vi "Omniax_mDrive_XYZR_MM_BR_RES.vi"() -> ()   [LabVIEW 2009]
uses:
  <vilib>/Instr/_visa.llb/VISA Configure Serial Port (Instr).vi
panel:
  out "R Backlash steps/sec":i32
  out "R Backlash":i32
  out "R Holding Current %":i32
  out "R Run Current %":i32
  out "R offset deg":dbl
  out "R deg/rev":dbl
  out "R steps/rev":u32
  out "R velocity PV step/sec":i32
  out "R MINPOS":i32=-94296
  out "R MAXPOS":i32=-34296
  out "R COM PORT":refnum<visa-resource-name>="COM5"
  in  "R Scan set":bool
  in  "R Scan Velocity SP deg/sec":dbl
  in  "R Scan Length SP deg":dbl
  in  "R Move Set":bool
  out "Reset R Motor Steps":i32
  in  "Reset R Position deg":dbl
  out "R Velocity MVdeg/sec":dbl
  in  "R Velocity SP deg/sec":dbl
  in  "R Position SP deg":dbl
  out "R Position MV deg":dbl
  out "R Scan velocity MV deg/sec":dbl format="%#_6f"
  out "R Scan length MV deg":dbl
  in  "R Scan Length SP steps":i32 min=-460800 max=460800 step=100
  in  "R Scan OK":bool
  in  "R Velocity SP step/sec":i32 min=1 max=102400
  in  "R Scan Velocity SP steps/sec":i32=1 min=1 max=102400 step=1
  in  "R Go":bool
  in  "R Step SP":i32=-20000 min=0 max=6144000 step=500
  out "R Position deg PV":dbl
  out "R Step PV":i32 max=2000
  out "R Backlash corr":bool
  out "R in Motion":bool
  out "R Scan":bool
  out "R in Range":bool
  out "Z COM PORT":refnum<visa-resource-name>="COM5"
  out "Z Backlash steps/sec":i32
  out "Z Backlash":i32
  out "Z Holding Current %":i32
  out "Z Run Current %":i32
  out "Z offset mm":dbl
  out "Z mm/rev":dbl
  out "Z steps/rev":u32
  out "Z  velocity PV step/sec":i32
  out "Z MINPOS":i32=-94296
  out "Z MAXPOS":i32=-34296
  in  "Z Scan set":bool
  in  "Z Scan Velocity SP mm/sec":dbl
  in  "Z Scan Length SP mm":dbl
  in  "Z Move Set":bool
  out "Reset Z Motor Steps":i32
  in  "Reset Z Position mm":dbl
  out "Z Velocity MV mm/sec":dbl
  in  "Z Velocity SP mm/sec":dbl
  in  "Z Position SP mm":dbl
  out "Z Position MV mm":dbl
  out "Z Scan velocity MV mm/sec":dbl format="%#_6f"
  out "Z Scan length MV mm":dbl
  in  "Z Scan Length SP steps":i32 min=-460800 max=460800 step=100
  in  "Z Scan OK":bool
  in  "Z Velocity SP step/sec":i32 min=1 max=102400
  in  "Z Scan Velocity SP steps/sec":i32=1 min=1 max=102400 step=1
  in  "Z Go":bool
  in  "Z Step SP":i32=-20000 min=0 max=2048000 step=500
  out "Z Position mm PV":dbl
  out "Z Step PV":i32 max=2000
  out "Z Backlash corr":bool
  out "Z in Motion":bool
  out "Z Scan":bool
  out "Z in Range":bool
  out "Reset X Motor Steps":i32
  in  "Reset X Position mm":dbl
  out "X Backlash corr":bool
  out "X  in Motion":bool
  out "X Scan":bool
  out "X  in Range":bool
  out "X Step PV":i32 max=2000
  out "X Position mm PV":dbl
  out "X velocity PV step/sec":i32
  in  "X Scan set":bool
  in  "X Scan Velocity SP mm/sec":dbl
  in  "X Scan Length SP mm":dbl
  in  "X Move Set":bool
  out "X Velocity MV mm/sec":dbl
  in  "X Velocity SP mm/sec":dbl
  in  "X Position SP mm":dbl
  out "X Position MV mm":dbl
  out "X Scan velocity MV mm/sec":dbl format="%#_6f"
  out "X Scan length MV mm":dbl
  in  "X Scan Length SP steps":i32 min=-460800 max=460800 step=100
  in  "X Scan OK":bool
  in  "X Velocity SP step/sec":i32 min=1 max=102400
  in  "X Scan Velocity SP steps/sec":i32=1 min=1 max=102400 step=1
  in  "X Go":bool
  in  "X Step SP":i32=-20000 min=-460800 max=460800 step=500
  out "X Backlash steps/sec":i32
  out "X Backlash":i32
  out "X Holding Current %":i32
  out "X Run Current %":i32
  out "X offset mm":dbl
  out "X mm/rev":dbl
  out "X steps/rev":u32
  out "X MAXPOS":i32=-34296
  out "X MINPOS":i32=-94296
  out "X COM PORT":refnum<visa-resource-name>="COM5"
  out "Y Backlash corr":bool
  in  "Y Scan set":bool
  in  "Y Scan Velocity SP mm/sec":dbl
  in  "Y Scan Length SP mm":dbl
  in  "Y Move Set":bool
  out "Y Backlash steps/sec":i32
  out "Y Backlash":i32
  out "Y in Motion":bool
  in  "Reset":bool
  out "Reset Y Motor Steps":i32
  in  "Reset Y Position mm":dbl
  out "Y Velocity MV mm/sec":dbl
  in  "Y Velocity SP mm/sec":dbl
  in  "Y Position SP mm":dbl
  out "Y Position MV mm":dbl
  out "Y Holding Current %":i32
  out "Y Run Current %":i32
  out "Y Scan velocity MV mm/sec":dbl format="%#_6f"
  out "Y Scan length MV mm":dbl
  in  "Scan Cancel":bool
  out "Y Position mm PV":dbl
  out "Y offset mm":dbl
  out "Y mm/rev":dbl
  out "Y steps/rev":u32
  out "Y velocity PV step/sec":i32
  in  "Y Scan Length SP steps":i32 min=-460800 max=460800 step=100
  out "Y Scan":bool
  in  "Y Scan OK":bool
  in  "Scan Go":bool
  in  "Y Velocity SP step/sec":i32 min=1 max=102400
  in  "Y Scan Velocity SP steps/sec":i32=1 min=1 max=102400 step=1
  in  "Stop":bool
  out "Y in Range":bool
  out "Y Step PV":i32 max=2000
  in  "Y Go":bool
  in  "Y Step SP":i32=-20000 min=-460800 max=460800 step=500
  out "Y MINPOS":i32=-94296
  out "Y MAXPOS":i32=-34296
  out "Y COM PORT":refnum<visa-resource-name>="COM5"
  # "LM"
  # "MV"
  # "BL"
  # "SC"
  # "MX"
  # "MY"
  # "MZ"
  # "MR"
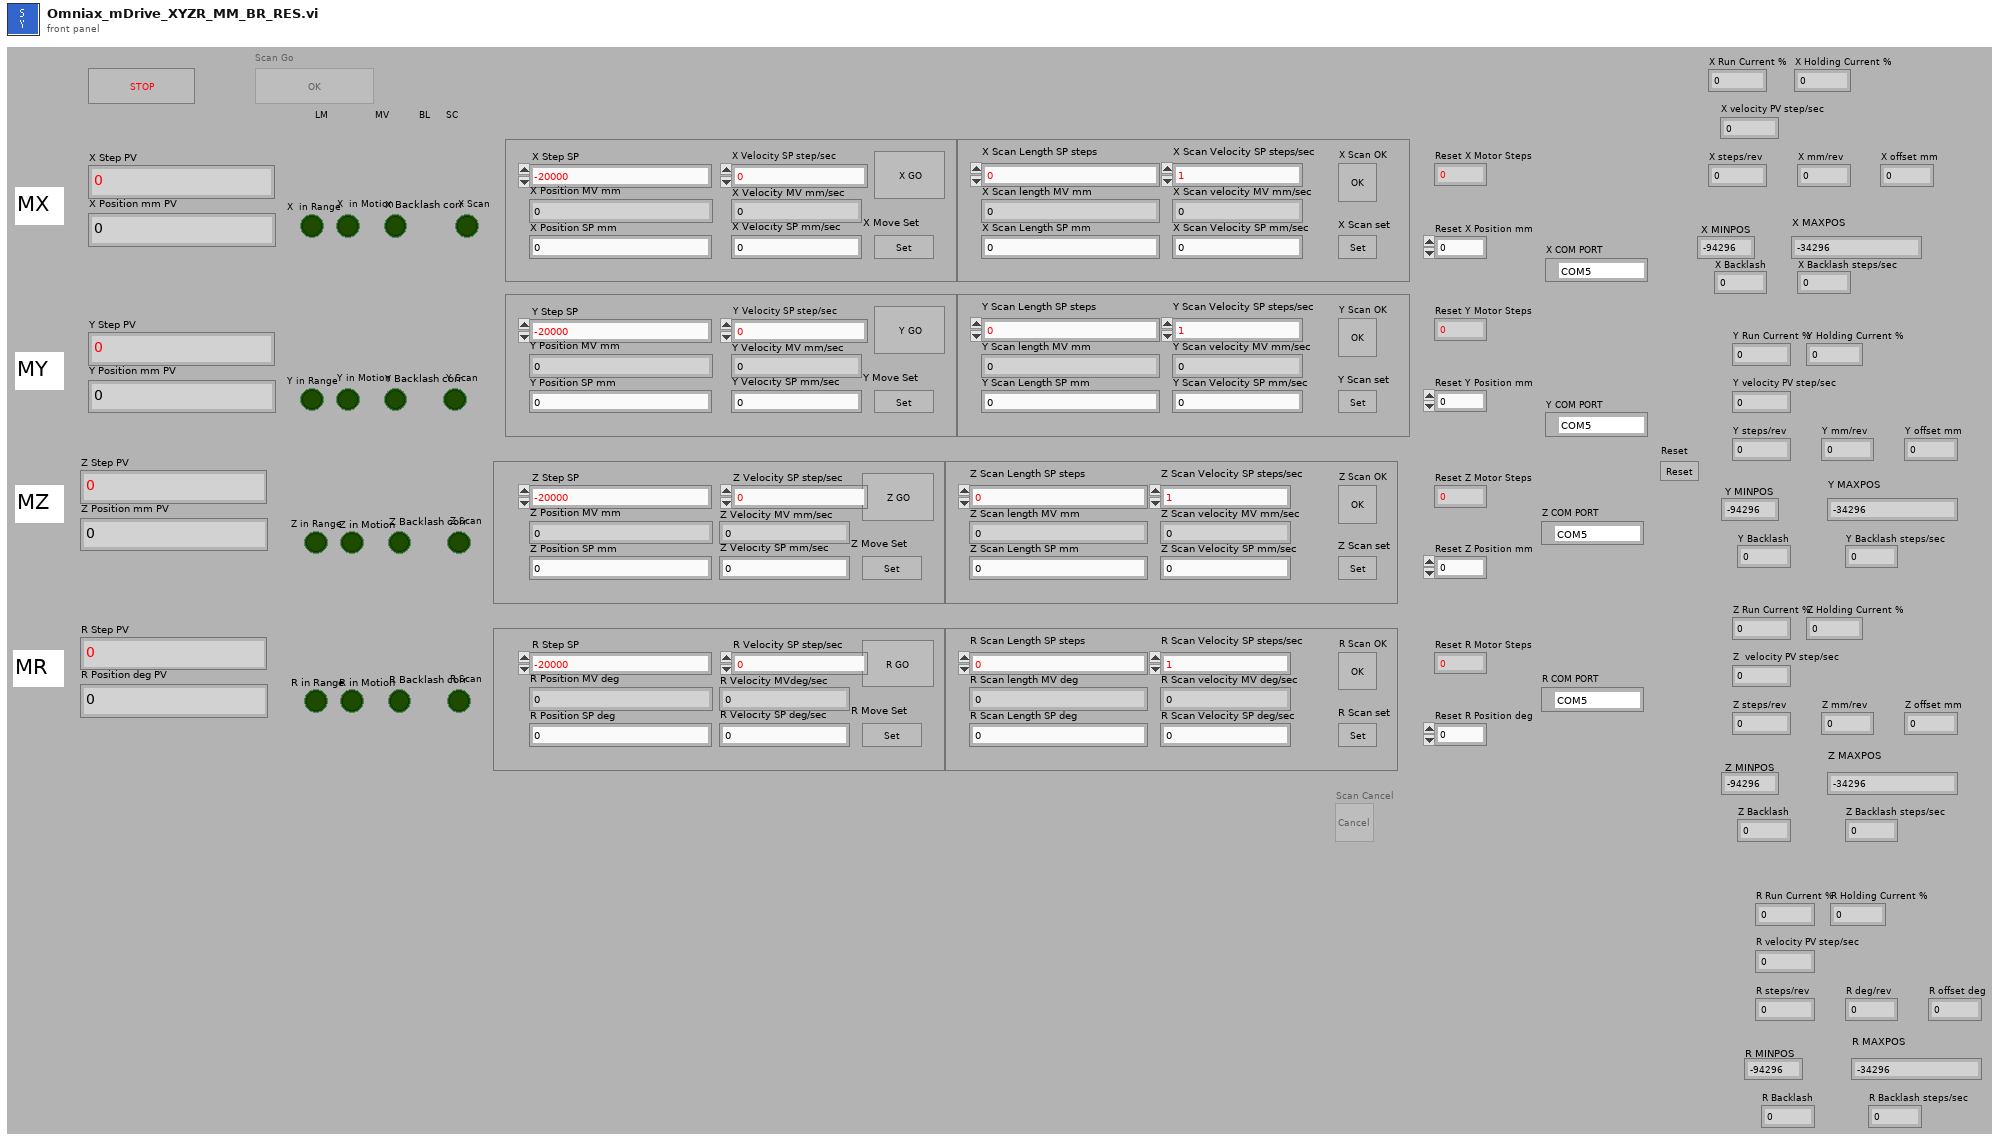
[diagram p1: front panel]
types:
  T1 = enum8{"Enabled", "Disabled", "Disabled and Grayed Out"}
  T2 = enum16{"Stop", "Reset", "Run Current", "Holding Current", "Accel Rate", "Decel Rate", "Move to Relative Position", "Move to Absolute Position", "Echo Mode", "Print Parameter", "Send String", "Microstep Resolution", "Set Current Position", "Max Velocity"}
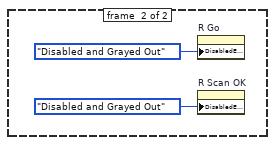
[diagram p2: hidden frame]
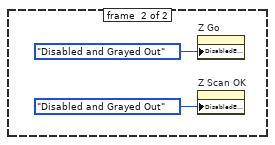
[diagram p5: hidden frame]
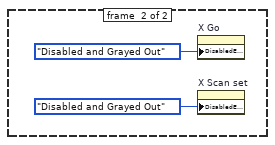
[diagram p8: hidden frame]
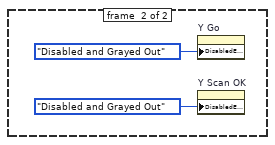
[diagram p11: hidden frame]
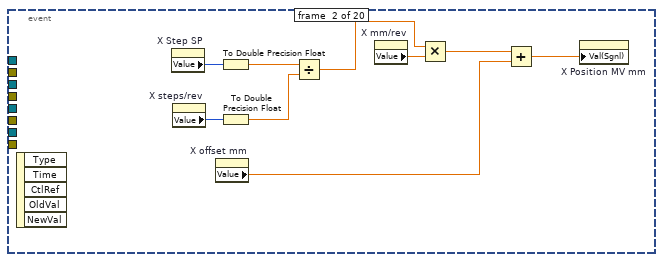
[diagram p14: hidden frame]
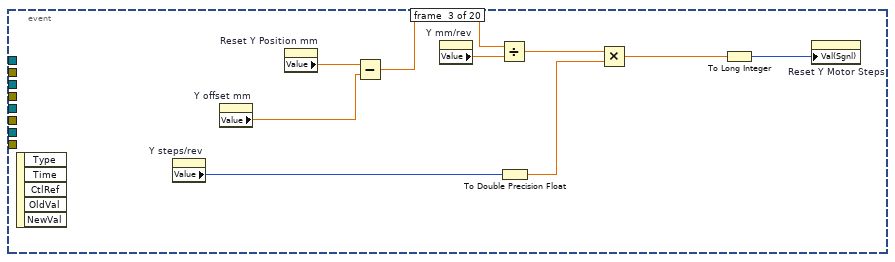
[diagram p15: hidden frame]
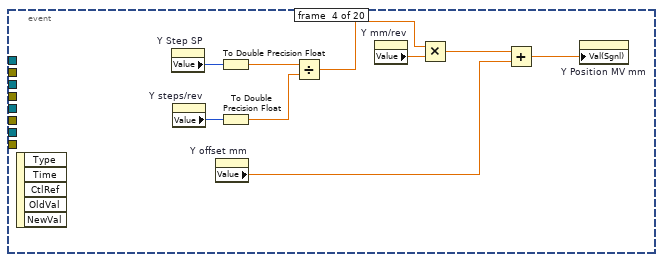
[diagram p16: hidden frame]
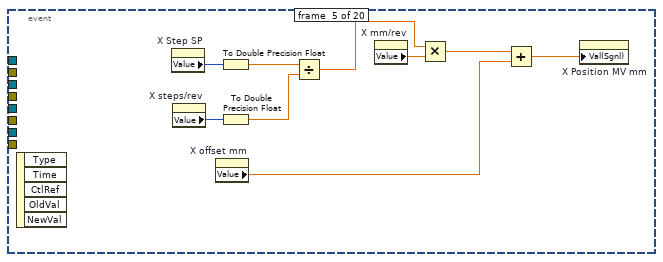
[diagram p17: hidden frame]
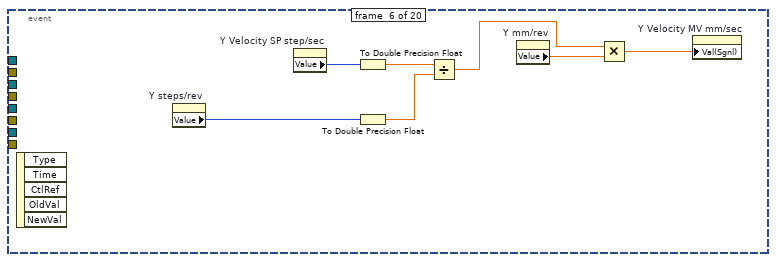
[diagram p18: hidden frame]
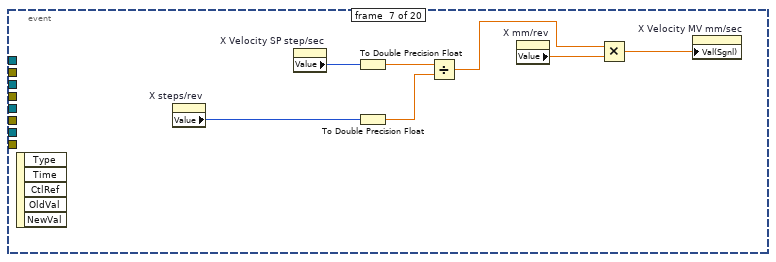
[diagram p19: hidden frame]
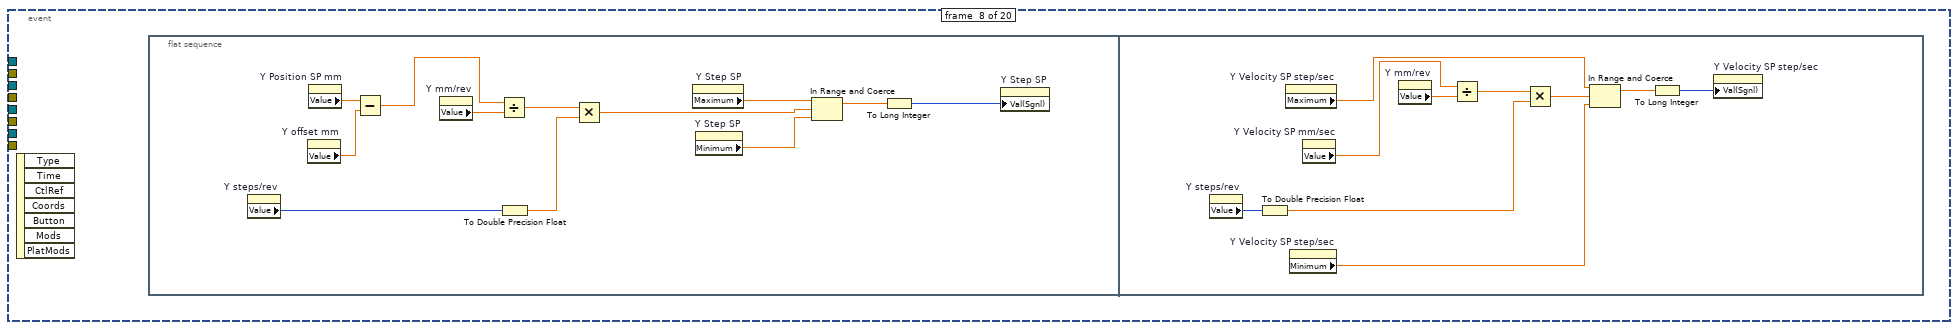
[diagram p20: hidden frame]
diagram:
  w11 = refnum<visa-resource-name> "COM11" ("COM PORT")
  w13 = u16 0 items=["None", "XON/XOFF", "RTS/CTS", "XON/XOFF & RTS/CTS", "DTR/DSR", "XON/XOFF & DTR/DSR"] ("flow control (0:none)")
  w14 = u16 10 items=["1.0"=10, "1.5"=15, "2.0"=20] ("stop bits (10: 1 bit)")
  w44 = refnum<visa-resource-name> "COM10" ("COM PORT")
  w46 = u16 0 items=["None", "XON/XOFF", "RTS/CTS", "XON/XOFF & RTS/CTS", "DTR/DSR", "XON/XOFF & DTR/DSR"] ("flow control (0:none)")
  w47 = u16 10 items=["1.0"=10, "1.5"=15, "2.0"=20] ("stop bits (10: 1 bit)")
  w57 = refnum<visa-resource-name> "COM8" ("COM PORT")
  w59 = u16 0 items=["None", "XON/XOFF", "RTS/CTS", "XON/XOFF & RTS/CTS", "DTR/DSR", "XON/XOFF & DTR/DSR"] ("flow control (0:none)")
  w60 = u16 10 items=["1.0"=10, "1.5"=15, "2.0"=20] ("stop bits (10: 1 bit)")
  w82 = refnum<visa-resource-name> "COM9" ("COM PORT")
  w84 = u16 0 items=["None", "XON/XOFF", "RTS/CTS", "XON/XOFF & RTS/CTS", "DTR/DSR", "XON/XOFF & DTR/DSR"] ("flow control (0:none)")
  w85 = u16 10 items=["1.0"=10, "1.5"=15, "2.0"=20] ("stop bits (10: 1 bit)")
  # "Stop bits"
  # "Stop bits"
  # "Stop bits"
  # "Stop bits"
  n1 = flat-sequence {
    frame #0 {
      w93 = 3.0 ("R deg/rev")
      w91 = u32 51200 ("step/rev")
      w95 = 102400 ("Value (Signaling)")
      n2 = property on="R Velocity SP step/sec" class="DigNum (strict)"("Val(Sgnl)"=w95) -> ()  [unwired: 2 in, 2 out]
      n3 = property on="R Velocity SP step/sec" class="DigNum (strict)"("Minimum"=1.0 ("Data Entry Limits:Minimum")) -> ()  [unwired: 2 in, 2 out]
      n4 = To Double Precision Float(number=w91) -> (double precision float=w92:dbl)
      n5 = To Double Precision Float(number=w95) -> (double precision float=w97:dbl)
      n6 = Divide(x=w97, y=w92) -> (x/y=w96:dbl)
      n7 = property on="R Velocity SP step/sec" class="DigNum (strict)"("Maximum"=w97) -> ()  [unwired: 2 in, 2 out]
      n8 = Multiply(x=w96, y=w93) -> (x*y=w94:dbl)
      n9 = property on="R Velocity SP deg/sec" class="DigNum (strict)"("Val(Sgnl)"=w94) -> ()  [unwired: 2 in, 2 out]
      "R offset deg" <- 0.0 ("R offset deg")
      "R deg/rev" <- w93
      "R steps/rev" <- w91
    }
  }
  n10 = flat-sequence {
    frame #0 {
      w100 = 1.0 ("MM/rev")
      w103 = u32 51200 ("step/rev")
      w98 = 102400 ("Value (Signaling)")
      n11 = property on="X Velocity SP step/sec" class="DigNum (strict)"("Minimum"=1.0 ("Data Entry Limits:Minimum")) -> ()  [unwired: 2 in, 2 out]
      n12 = property on="X Velocity SP step/sec" class="DigNum (strict)"("Val(Sgnl)"=w98) -> ()  [unwired: 2 in, 2 out]
      n13 = To Double Precision Float(number=w103) -> (double precision float=w102:dbl)
      n14 = To Double Precision Float(number=w98) -> (double precision float=w104:dbl)
      n15 = Divide(x=w104, y=w102) -> (x/y=w99:dbl)
      n16 = property on="X Velocity SP step/sec" class="DigNum (strict)"("Maximum"=w104) -> ()  [unwired: 2 in, 2 out]
      n17 = Multiply(x=w99, y=w100) -> (x*y=w101:dbl)
      n18 = property on="X Velocity SP mm/sec" class="DigNum (strict)"("Val(Sgnl)"=w101) -> ()  [unwired: 2 in, 2 out]
      "X offset mm" <- 0.0 ("offset")
      "X steps/rev" <- w103
      "X mm/rev" <- w100
    }
  }
  n19 = flat-sequence {
    frame #0 {
      w108 = 1.0 ("Z mm/rev")
      w107 = u32 51200 ("step/rev")
      w109 = 102400 ("Value (Signaling)")
      n20 = property on="Z Velocity SP step/sec" class="DigNum (strict)"("Val(Sgnl)"=w109) -> ()  [unwired: 2 in, 2 out]
      n21 = property on="Z Velocity SP step/sec" class="DigNum (strict)"("Minimum"=1.0 ("Data Entry Limits:Minimum")) -> ()  [unwired: 2 in, 2 out]
      n22 = To Double Precision Float(number=w107) -> (double precision float=w112:dbl)
      n23 = To Double Precision Float(number=w109) -> (double precision float=w113:dbl)
      n24 = Divide(x=w113, y=w112) -> (x/y=w110:dbl)
      n25 = property on="Z Velocity SP step/sec" class="DigNum (strict)"("Maximum"=w113) -> ()  [unwired: 2 in, 2 out]
      n26 = Multiply(x=w110, y=w108) -> (x*y=w111:dbl)
      n27 = property on="Z Velocity SP mm/sec" class="DigNum (strict)"("Val(Sgnl)"=w111) -> ()  [unwired: 2 in, 2 out]
      "Z offset mm" <- 0.0 ("Z offset mm")
      "Z mm/rev" <- w108
      "Z steps/rev" <- w107
    }
  }
  n28 = flat-sequence {
    frame #0 {
      n29 = property on="X Backlash corr" class="Bool (strict)"("Val(Sgnl)"=FALSE ("Value (Signaling)")) -> ()  [unwired: 2 in, 2 out]
      n30 = property on="Z Backlash corr" class="Bool (strict)"("Val(Sgnl)"=FALSE ("Value (Signaling)")) -> ()  [unwired: 2 in, 2 out]
      n31 = property on="Y Backlash corr" class="Bool (strict)"("Val(Sgnl)"=FALSE ("Value (Signaling)")) -> ()  [unwired: 2 in, 2 out]
      n32 = property on="R Backlash corr" class="Bool (strict)"("Val(Sgnl)"=FALSE ("Value (Signaling)")) -> ()  [unwired: 2 in, 2 out]
      "Z Backlash steps/sec" <- 25600 ("Z Backlash steps/sec")
      "Z Backlash" <- -12800 ("Z Backlash")
      "X Backlash steps/sec" <- 25600 ("Value (Signaling)")
      "X Backlash" <- -5120 ("Backlash2")
      "Y Backlash" <- -5120 ("Backlash2")
      "Y Backlash steps/sec" <- 25600 ("Value (Signaling)")
      "R Backlash steps/sec" <- 25600 ("R Backlash steps/sec")
      "R Backlash" <- -12800 ("R Backlash")
    }
  }
  n33 = flat-sequence {
    frame #0 {
      "Z Holding Current %" <- 25 ("Z Holding Current %")
      "Z Run Current %" <- 60 ("Z Run Current %")
      "X Run Current %" <- 60 ("Run Current %")
      "X Holding Current %" <- 25 ("Holding Current %")
      "Y Run Current %" <- 60 ("Run Current %")
      "Y Holding Current %" <- 25 ("Holding Current %")
      "R Holding Current %" <- 25 ("R Holding Current %")
      "R Run Current %" <- 60 ("R Run Current %")
    }
  }
  n34 = flat-sequence {
    frame #0 {
      n35 = property on="Y Scan" class="Bool (strict)"("Val(Sgnl)"=FALSE ("Value (Signaling)")) -> ()  [unwired: 2 in, 2 out]
      n36 = property on="Y Scan Velocity SP mm/sec" class="DigNum (strict)"("Val(Sgnl)"=0.1 ("Value (Signaling)")) -> ()  [unwired: 2 in, 2 out]
      n37 = property on="Z Scan Velocity SP mm/sec" class="DigNum (strict)"("Val(Sgnl)"=0.1 ("Value (Signaling)")) -> ()  [unwired: 2 in, 2 out]
      n38 = property on="R Scan" class="Bool (strict)"("Val(Sgnl)"=FALSE ("Value (Signaling)")) -> ()  [unwired: 2 in, 2 out]
      n39 = property on="Z Scan" class="Bool (strict)"("Val(Sgnl)"=FALSE ("Value (Signaling)")) -> ()  [unwired: 2 in, 2 out]
      n40 = property on="R Velocity SP deg/sec" class="DigNum (strict)"("Val(Sgnl)"=0.1 ("Value (Signaling)")) -> ()  [unwired: 2 in, 2 out]
      n41 = property on="X Scan" class="Bool (strict)"("Val(Sgnl)"=FALSE ("Value (Signaling)")) -> ()  [unwired: 2 in, 2 out]
      n42 = property on="X Scan Velocity SP mm/sec" class="DigNum (strict)"("Val(Sgnl)"=0.1 ("Value (Signaling)")) -> ()  [unwired: 2 in, 2 out]
      n43 = property on="Scan Go" class="Bool"("DisabledEnum"=T1."Disabled and Grayed Out" ("Disabled")) -> ()  [unwired: 2 in, 2 out]
      n44 = property on="Scan Cancel" class="Bool"("DisabledEnum"=T1."Disabled and Grayed Out" ("Disabled")) -> ()  [unwired: 2 in, 2 out]
    }
  }
  n45 = flat-sequence {
    frame #0 {
      w148 = 1.0 ("MM/rev")
      w151 = u32 51200 ("step/rev")
      w146 = 102400 ("Value (Signaling)")
      n46 = property on="Y Velocity SP step/sec" class="DigNum (strict)"("Minimum"=1.0 ("Data Entry Limits:Minimum")) -> ()  [unwired: 2 in, 2 out]
      n47 = property on="Y Velocity SP step/sec" class="DigNum (strict)"("Val(Sgnl)"=w146) -> ()  [unwired: 2 in, 2 out]
      n48 = To Double Precision Float(number=w151) -> (double precision float=w150:dbl)
      n49 = To Double Precision Float(number=w146) -> (double precision float=w152:dbl)
      n50 = Divide(x=w152, y=w150) -> (x/y=w147:dbl)
      n51 = property on="Y Velocity SP step/sec" class="DigNum (strict)"("Maximum"=w152) -> ()  [unwired: 2 in, 2 out]
      n52 = Multiply(x=w147, y=w148) -> (x*y=w149:dbl)
      n53 = property on="Y Velocity SP mm/sec" class="DigNum (strict)"("Val(Sgnl)"=w149) -> ()  [unwired: 2 in, 2 out]
      "Y offset mm" <- 0.0 ("offset")
      "Y steps/rev" <- w151
      "Y mm/rev" <- w148
    }
  }
  n54 = call-poly "VISA Configure Serial Port"("VISA resource name"=w82, "timeout (10sec)"=u32 10000, "baud rate (9600)"=u32 9600, "data bits (8)"=u16 8, "parity (0:none)"=enum16{"None", "Odd", "Even", "Mark", "Space"}."None", "stop bits (10: 1 bit)"=w85, "flow control (0:none)"=w84) -> ("VISA resource name out"=w75:refnum<visa-resource-name>, "error out"=w74:errorcluster)  [unwired: 7 in]
  n55 = flat-sequence {
    tunnel: w74 -> [w161]
    tunnel: w75 -> [w159]
    tunnel: [w158] -> w73
    tunnel: [w160] -> w71
    tunnel: w73 -> [w168]
    tunnel: [w167] -> w72
    tunnel: w71 -> [w165]
    tunnel: [w166] -> w70
    tunnel: [w178] -> w77
    tunnel: [w179] -> w76
    tunnel: w72 -> [w177]
    tunnel: w70 -> [w176]
    tunnel: w77 -> [w189]
    tunnel: w76 -> [w188]
    tunnel: [w191] -> w43
    tunnel: [w190] -> w42
    tunnel: [w185] -> w41
    tunnel: [w196] -> w80
    tunnel: [w197] -> w81
    tunnel: w43 -> [w197]
    tunnel: w42 -> [w196]
    tunnel: w41 -> [w192]
    frame #0 {
      # "Run Current %"
      n56 = property on="Y Run Current %" class="DigNum (strict)"() -> ("Value"=w156:i32)  [unwired: 2 in, 2 out]
      n57 = Number To Decimal String(number=w156) -> (decimal integer string=w157:string)  [unwired: 1 in]
      n58 = call "mDrive Send Command.vi"("error in (no error)"=w161, "Extra"=w157, "Command"=T2."Run Current", "VISA resource name"=w159) -> ("error out"=w160:errorcluster, "VISA resource name out"=w158:refnum<visa-resource-name>)  [unwired: 3 in, 1 out]
    }
    frame #1 {
      # "Holding Current %"
      n59 = property on="Y Holding Current %" class="DigNum (strict)"() -> ("Value"=w163:i32)  [unwired: 2 in, 2 out]
      n60 = Number To Decimal String(number=w163) -> (decimal integer string=w164:string)  [unwired: 1 in]
      n61 = call "mDrive Send Command.vi"("error in (no error)"=w165, "Extra"=w164, "Command"=T2."Holding Current", "VISA resource name"=w168) -> ("error out"=w166:errorcluster, "VISA resource name out"=w167:refnum<visa-resource-name>)  [unwired: 3 in, 1 out]
    }
    frame #2 {
      # "Print Velocity Ma"
      # "Velocity Max"
      n62 = property on="Y Velocity SP step/sec" class="DigNum (strict)"() -> ("Value"=w175:i32)  [unwired: 2 in, 2 out]
      n63 = Number To Decimal String(number=w175) -> (decimal integer string=w174:string)  [unwired: 1 in]
      n64 = call "mDrive Send Command.vi"("error in (no error)"=w176, "Extra"=w174, "Command"=T2."Max Velocity", "VISA resource name"=w177) -> ("error out"=w172:errorcluster, "VISA resource name out"=w182:refnum<visa-resource-name>)  [unwired: 3 in, 1 out]
      n65 = call "mDrive Send Command.vi"("error in (no error)"=w172, "Extra"="VM", "Command"=T2."Print Parameter", "VISA resource name"=w182) -> ("error out"=w179:errorcluster, "read buffer"=w180:string, "VISA resource name out"=w178:refnum<visa-resource-name>)  [unwired: 3 in]
      n66 = Decimal String To Number(string=w180, offset=0) -> (number=w173:i32)  [unwired: 1 in, 1 out]
      n67 = property on="Y scan velocity MV step/sec" class="DigNum (strict)"("Val(Sgnl)"=w173) -> ()  [unwired: 2 in, 2 out]
    }
    frame #3 {
      # "PRINT POSITION"
      n68 = call "mDrive Send Command.vi"("error in (no error)"=w188, "Extra"="P", "Command"=T2."Print Parameter", "VISA resource name"=w189) -> ("error out"=w190:errorcluster, "read buffer"=w187:string, "VISA resource name out"=w191:refnum<visa-resource-name>)  [unwired: 3 in]
      n69 = Decimal String To Number(string=w187, offset=0) -> (number=w185:i32)  [unwired: 1 in, 1 out]
    }
    frame #4 {
      w194 = -460800 ("lower limit")
      w195 = 460800 ("upper limit")
      n70 = property on="Y Step SP" class="DigNum (strict)"("Val(Sgnl)"=w192) -> ()  [unwired: 2 in, 2 out]
      n71 = property on="Y Step SP" class="DigNum (strict)"("Maximum"=w195) -> ()  [unwired: 2 in, 2 out]
      n72 = property on="Y Step SP" class="DigNum (strict)"("Minimum"=w194) -> ()  [unwired: 2 in, 2 out]
      n73 = In Range and Coerce(upper limit=w195, x=w192, lower limit=w194) -> (In Range?=w193:bool)  [unwired: 1 out]
      n74 = property on="Y in Range" class="Bool (strict)"("Val(Sgnl)"=w193) -> ()  [unwired: 2 in, 2 out]
      "Y MINPOS" <- w194
      "Y MAXPOS" <- w195
    }
  }
  n75 = call-poly "VISA Configure Serial Port"("VISA resource name"=w57, "timeout (10sec)"=u32 10000, "baud rate (9600)"=u32 9600, "data bits (8)"=u16 8, "parity (0:none)"=enum16{"None", "Odd", "Even", "Mark", "Space"}."None", "stop bits (10: 1 bit)"=w60, "flow control (0:none)"=w59) -> ("VISA resource name out"=w56:refnum<visa-resource-name>, "error out"=w55:errorcluster)  [unwired: 7 in]
  n76 = call-poly "VISA Configure Serial Port"("VISA resource name"=w11, "timeout (10sec)"=u32 10000, "baud rate (9600)"=u32 9600, "data bits (8)"=u16 8, "parity (0:none)"=enum16{"None", "Odd", "Even", "Mark", "Space"}."None", "stop bits (10: 1 bit)"=w14, "flow control (0:none)"=w13) -> ("VISA resource name out"=w10:refnum<visa-resource-name>, "error out"=w9:errorcluster)  [unwired: 7 in]
  n77 = call-poly "VISA Configure Serial Port"("VISA resource name"=w44, "timeout (10sec)"=u32 10000, "baud rate (9600)"=u32 9600, "data bits (8)"=u16 8, "parity (0:none)"=enum16{"None", "Odd", "Even", "Mark", "Space"}."None", "stop bits (10: 1 bit)"=w47, "flow control (0:none)"=w46) -> ("VISA resource name out"=w28:refnum<visa-resource-name>, "error out"=w27:errorcluster)  [unwired: 7 in]
  n78 = flat-sequence {
    tunnel: w55 -> [w204]
    tunnel: w56 -> [w202]
    tunnel: [w201] -> w69
    tunnel: [w203] -> w68
    tunnel: w69 -> [w211]
    tunnel: [w210] -> w67
    tunnel: w68 -> [w208]
    tunnel: [w209] -> w66
    tunnel: [w221] -> w65
    tunnel: [w222] -> w64
    tunnel: w67 -> [w220]
    tunnel: w66 -> [w219]
    tunnel: w65 -> [w232]
    tunnel: w64 -> [w231]
    tunnel: [w234] -> w40
    tunnel: [w233] -> w39
    tunnel: [w228] -> w38
    tunnel: [w239] -> w53
    tunnel: [w240] -> w54
    tunnel: w40 -> [w240]
    tunnel: w39 -> [w239]
    tunnel: w38 -> [w235]
    frame #0 {
      # "Run Current %"
      n79 = property on="X Run Current %" class="DigNum (strict)"() -> ("Value"=w199:i32)  [unwired: 2 in, 2 out]
      n80 = Number To Decimal String(number=w199) -> (decimal integer string=w200:string)  [unwired: 1 in]
      n81 = call "mDrive Send Command.vi"("error in (no error)"=w204, "Extra"=w200, "Command"=T2."Run Current", "VISA resource name"=w202) -> ("error out"=w203:errorcluster, "VISA resource name out"=w201:refnum<visa-resource-name>)  [unwired: 3 in, 1 out]
    }
    frame #1 {
      # "Holding Current %"
      n82 = property on="X Holding Current %" class="DigNum (strict)"() -> ("Value"=w206:i32)  [unwired: 2 in, 2 out]
      n83 = Number To Decimal String(number=w206) -> (decimal integer string=w207:string)  [unwired: 1 in]
      n84 = call "mDrive Send Command.vi"("error in (no error)"=w208, "Extra"=w207, "Command"=T2."Holding Current", "VISA resource name"=w211) -> ("error out"=w209:errorcluster, "VISA resource name out"=w210:refnum<visa-resource-name>)  [unwired: 3 in, 1 out]
    }
    frame #2 {
      # "Print Velocity Ma"
      # "Velocity Max"
      n85 = property on="X Velocity SP step/sec" class="DigNum (strict)"() -> ("Value"=w218:i32)  [unwired: 2 in, 2 out]
      n86 = Number To Decimal String(number=w218) -> (decimal integer string=w217:string)  [unwired: 1 in]
      n87 = call "mDrive Send Command.vi"("error in (no error)"=w219, "Extra"=w217, "Command"=T2."Max Velocity", "VISA resource name"=w220) -> ("error out"=w215:errorcluster, "VISA resource name out"=w225:refnum<visa-resource-name>)  [unwired: 3 in, 1 out]
      n88 = call "mDrive Send Command.vi"("error in (no error)"=w215, "Extra"="VM", "Command"=T2."Print Parameter", "VISA resource name"=w225) -> ("error out"=w222:errorcluster, "read buffer"=w223:string, "VISA resource name out"=w221:refnum<visa-resource-name>)  [unwired: 3 in]
      n89 = Decimal String To Number(string=w223, offset=0) -> (number=w216:i32)  [unwired: 1 in, 1 out]
      n90 = property on="X velocity PV step/sec" class="DigNum (strict)"("Val(Sgnl)"=w216) -> ()  [unwired: 2 in, 2 out]
    }
    frame #3 {
      # "PRINT POSITION"
      n91 = call "mDrive Send Command.vi"("error in (no error)"=w231, "Extra"="P", "Command"=T2."Print Parameter", "VISA resource name"=w232) -> ("error out"=w233:errorcluster, "read buffer"=w230:string, "VISA resource name out"=w234:refnum<visa-resource-name>)  [unwired: 3 in]
      n92 = Decimal String To Number(string=w230, offset=0) -> (number=w228:i32)  [unwired: 1 in, 1 out]
    }
    frame #4 {
      w237 = -460800 ("lower limit")
      w238 = 460800 ("upper limit")
      n93 = property on="X Step SP" class="DigNum (strict)"("Val(Sgnl)"=w235) -> ()  [unwired: 2 in, 2 out]
      n94 = property on="X Step SP" class="DigNum (strict)"("Maximum"=w238) -> ()  [unwired: 2 in, 2 out]
      n95 = property on="X Step SP" class="DigNum (strict)"("Minimum"=w237) -> ()  [unwired: 2 in, 2 out]
      n96 = In Range and Coerce(upper limit=w238, x=w235, lower limit=w237) -> (In Range?=w236:bool)  [unwired: 1 out]
      n97 = property on="X  in Range" class="Bool (strict)"("Val(Sgnl)"=w236) -> ()  [unwired: 2 in, 2 out]
      "X MINPOS" <- w237
      "X MAXPOS" <- w238
    }
  }
  n98 = flat-sequence {
    tunnel: w10 -> [w246]
    tunnel: [w245] -> w26
    tunnel: [w247] -> w25
    tunnel: w9 -> [w241]
    tunnel: w26 -> [w254]
    tunnel: [w253] -> w24
    tunnel: w25 -> [w251]
    tunnel: [w252] -> w23
    tunnel: [w264] -> w22
    tunnel: [w265] -> w21
    tunnel: w24 -> [w263]
    tunnel: w23 -> [w262]
    tunnel: w22 -> [w275]
    tunnel: w21 -> [w274]
    tunnel: [w277] -> w20
    tunnel: [w276] -> w19
    tunnel: [w271] -> w18
    tunnel: [w282] -> w3
    tunnel: [w283] -> w4
    tunnel: w20 -> [w283]
    tunnel: w19 -> [w282]
    tunnel: w18 -> [w280]
    frame #0 {
      # "Run Current %"
      n99 = property on="R Run Current %" class="DigNum (strict)"() -> ("Value"=w243:i32)  [unwired: 2 in, 2 out]
      n100 = Number To Decimal String(number=w243) -> (decimal integer string=w244:string)  [unwired: 1 in]
      n101 = call "mDrive Send Command.vi"("error in (no error)"=w241, "Extra"=w244, "Command"=T2."Run Current", "VISA resource name"=w246) -> ("error out"=w247:errorcluster, "VISA resource name out"=w245:refnum<visa-resource-name>)  [unwired: 3 in, 1 out]
    }
    frame #1 {
      # "Holding Current %"
      n102 = property on="R Holding Current %" class="DigNum (strict)"() -> ("Value"=w249:i32)  [unwired: 2 in, 2 out]
      n103 = Number To Decimal String(number=w249) -> (decimal integer string=w250:string)  [unwired: 1 in]
      n104 = call "mDrive Send Command.vi"("error in (no error)"=w251, "Extra"=w250, "Command"=T2."Holding Current", "VISA resource name"=w254) -> ("error out"=w252:errorcluster, "VISA resource name out"=w253:refnum<visa-resource-name>)  [unwired: 3 in, 1 out]
    }
    frame #2 {
      # "Print Velocity Ma"
      # "Velocity Max"
      n105 = property on="R Velocity SP step/sec" class="DigNum (strict)"() -> ("Value"=w261:i32)  [unwired: 2 in, 2 out]
      n106 = Number To Decimal String(number=w261) -> (decimal integer string=w260:string)  [unwired: 1 in]
      n107 = call "mDrive Send Command.vi"("error in (no error)"=w262, "Extra"=w260, "Command"=T2."Max Velocity", "VISA resource name"=w263) -> ("error out"=w258:errorcluster, "VISA resource name out"=w268:refnum<visa-resource-name>)  [unwired: 3 in, 1 out]
      n108 = call "mDrive Send Command.vi"("error in (no error)"=w258, "Extra"="VM", "Command"=T2."Print Parameter", "VISA resource name"=w268) -> ("error out"=w265:errorcluster, "read buffer"=w266:string, "VISA resource name out"=w264:refnum<visa-resource-name>)  [unwired: 3 in]
      n109 = Decimal String To Number(string=w266, offset=0) -> (number=w259:i32)  [unwired: 1 in, 1 out]
      n110 = property on="R velocity PV step/sec" class="DigNum (strict)"("Val(Sgnl)"=w259) -> ()  [unwired: 2 in, 2 out]
    }
    frame #3 {
      # "PRINT POSITION"
      n111 = call "mDrive Send Command.vi"("error in (no error)"=w274, "Extra"="P", "Command"=T2."Print Parameter", "VISA resource name"=w275) -> ("error out"=w276:errorcluster, "read buffer"=w273:string, "VISA resource name out"=w277:refnum<visa-resource-name>)  [unwired: 3 in]
      n112 = Decimal String To Number(string=w273, offset=0) -> (number=w271:i32)  [unwired: 1 in, 1 out]
    }
    frame #4 {
      w279 = 0 ("lower limit")
      w278 = 6144000 ("upper limit")
      n113 = property on="R Step SP" class="DigNum (strict)"("Val(Sgnl)"=w280) -> ()  [unwired: 2 in, 2 out]
      n114 = property on="R Step SP" class="DigNum (strict)"("Maximum"=w278) -> ()  [unwired: 2 in, 2 out]
      n115 = property on="R Step SP" class="DigNum (strict)"("Minimum"=w279) -> ()  [unwired: 2 in, 2 out]
      n116 = In Range and Coerce(upper limit=w278, x=w280, lower limit=w279) -> (In Range?=w281:bool)  [unwired: 1 out]
      n117 = property on="R in Range" class="Bool (strict)"("Val(Sgnl)"=w281) -> ()  [unwired: 2 in, 2 out]
      "R MINPOS" <- w279
      "R MAXPOS" <- w278
    }
  }
  n118 = flat-sequence {
    tunnel: w27 -> [w290]
    tunnel: w28 -> [w288]
    tunnel: [w287] -> w37
    tunnel: [w289] -> w36
    tunnel: w37 -> [w297]
    tunnel: [w296] -> w35
    tunnel: w36 -> [w294]
    tunnel: [w295] -> w34
    tunnel: [w307] -> w33
    tunnel: [w308] -> w32
    tunnel: w35 -> [w306]
    tunnel: w34 -> [w305]
    tunnel: w33 -> [w318]
    tunnel: w32 -> [w317]
    tunnel: [w320] -> w31
    tunnel: [w319] -> w30
    tunnel: [w314] -> w29
    tunnel: [w325] -> w7
    tunnel: [w326] -> w8
    tunnel: w31 -> [w326]
    tunnel: w30 -> [w325]
    tunnel: w29 -> [w323]
    frame #0 {
      # "Run Current %"
      n119 = property on="Z Run Current %" class="DigNum (strict)"() -> ("Value"=w285:i32)  [unwired: 2 in, 2 out]
      n120 = Number To Decimal String(number=w285) -> (decimal integer string=w286:string)  [unwired: 1 in]
      n121 = call "mDrive Send Command.vi"("error in (no error)"=w290, "Extra"=w286, "Command"=T2."Run Current", "VISA resource name"=w288) -> ("error out"=w289:errorcluster, "VISA resource name out"=w287:refnum<visa-resource-name>)  [unwired: 3 in, 1 out]
    }
    frame #1 {
      # "Holding Current %"
      n122 = property on="Z Run Current %" class="DigNum (strict)"() -> ("Value"=w292:i32)  [unwired: 2 in, 2 out]
      n123 = Number To Decimal String(number=w292) -> (decimal integer string=w293:string)  [unwired: 1 in]
      n124 = call "mDrive Send Command.vi"("error in (no error)"=w294, "Extra"=w293, "Command"=T2."Holding Current", "VISA resource name"=w297) -> ("error out"=w295:errorcluster, "VISA resource name out"=w296:refnum<visa-resource-name>)  [unwired: 3 in, 1 out]
    }
    frame #2 {
      # "Print Velocity Ma"
      # "Velocity Max"
      n125 = property on="Z Velocity SP step/sec" class="DigNum (strict)"() -> ("Value"=w304:i32)  [unwired: 2 in, 2 out]
      n126 = Number To Decimal String(number=w304) -> (decimal integer string=w303:string)  [unwired: 1 in]
      n127 = call "mDrive Send Command.vi"("error in (no error)"=w305, "Extra"=w303, "Command"=T2."Max Velocity", "VISA resource name"=w306) -> ("error out"=w301:errorcluster, "VISA resource name out"=w311:refnum<visa-resource-name>)  [unwired: 3 in, 1 out]
      n128 = call "mDrive Send Command.vi"("error in (no error)"=w301, "Extra"="VM", "Command"=T2."Print Parameter", "VISA resource name"=w311) -> ("error out"=w308:errorcluster, "read buffer"=w309:string, "VISA resource name out"=w307:refnum<visa-resource-name>)  [unwired: 3 in]
      n129 = Decimal String To Number(string=w309, offset=0) -> (number=w302:i32)  [unwired: 1 in, 1 out]
      n130 = property on="Z  velocity PV step/sec" class="DigNum (strict)"("Val(Sgnl)"=w302) -> ()  [unwired: 2 in, 2 out]
    }
    frame #3 {
      # "PRINT POSITION"
      n131 = call "mDrive Send Command.vi"("error in (no error)"=w317, "Extra"="P", "Command"=T2."Print Parameter", "VISA resource name"=w318) -> ("error out"=w319:errorcluster, "read buffer"=w316:string, "VISA resource name out"=w320:refnum<visa-resource-name>)  [unwired: 3 in]
      n132 = Decimal String To Number(string=w316, offset=0) -> (number=w314:i32)  [unwired: 1 in, 1 out]
    }
    frame #4 {
      w321 = 0 ("lower limit")
      w322 = 2048000 ("upper limit")
      n133 = property on="Z Step SP" class="DigNum (strict)"("Val(Sgnl)"=w323) -> ()  [unwired: 2 in, 2 out]
      n134 = property on="Z Step SP" class="DigNum (strict)"("Maximum"=w322) -> ()  [unwired: 2 in, 2 out]
      n135 = property on="Z Step SP" class="DigNum (strict)"("Minimum"=w321) -> ()  [unwired: 2 in, 2 out]
      n136 = In Range and Coerce(upper limit=w322, x=w323, lower limit=w321) -> (In Range?=w324:bool)  [unwired: 1 out]
      n137 = property on="Z in Range" class="Bool (strict)"("Val(Sgnl)"=w324) -> ()  [unwired: 2 in, 2 out]
      "Z MINPOS" <- w321
      "Z MAXPOS" <- w322
    }
  }
  n138 = while {
    tunnel: w81 -> [w340]
    tunnel: w80 -> [w343]
    tunnel: [w344] -> w78
    tunnel: [w342] -> w79
    tunnel: w54 -> [w338]
    tunnel: w53 -> [w337]
    tunnel: [w336] -> w52
    tunnel: [w335] -> w51
    tunnel: w8 -> [w334]
    tunnel: w7 -> [w333]
    tunnel: [w332] -> w6
    tunnel: [w331] -> w5
    tunnel: w4 -> [w330]
    tunnel: w3 -> [w329]
    tunnel: [w328] -> w2
    tunnel: [w327] -> w1
    stop <- w339 stop-if-true
    n139 = flat-sequence {
      frame #0 {
      }
    }
    n140 = flat-sequence {
      frame #0 {
      }
    }
    n141 = flat-sequence {
      frame #0 {
      }
    }
    n142 = flat-sequence {
      frame #0 {
      }
    }
    n143 = flat-sequence {
      frame #0 {
      }
    }
    n144 = event shown="[16] \"Stop\": Mouse Down" {
      selector: _ -> [_ _ _ _ _ _ _ _ _ _ _ _ _ _ _ _ _ _ _ _]
      dyn-events: _ -> [_ _ _ _ _ _ _ _ _ _ _ _ _ _ _ _ _ _ _ _]
      timeout: 500 -> [_ _ _ _ _ _ _ _ _ _ _ _ _ _ _ _ _ _ _ _]
      tunnel: w343 -> [w412 _ _ _ _ _ _ _ _ _ _ w1143 _ _ w1287 w1316 w1332 w1370 w1429 w1487]
      tunnel: [w411 _ _ _ _ _ _ _ _ _ _ w1149 _ _ w1285 w1316 w1330 w1372 w1426 w1485] -> w344
      tunnel: w340 -> [w409 _ _ _ _ _ _ _ _ _ _ w1144 _ _ w1286 w1317 w1333 w1371 w1428 w1488]
      tunnel: [w410 _ _ _ _ _ _ _ _ _ _ w1150 _ _ w1282 w1317 w1331 w1373 w1427 w1486] -> w342
      tunnel: [_ _ _ _ _ _ _ _ _ _ _ _ _ _ _ TRUE _ _ _ _] -> w339
      tunnel: w338 -> [w382 _ _ _ _ _ _ _ _ _ _ _ w1195 w1250 _ _ w1327 w1363 _ w1484]
      tunnel: w337 -> [w381 _ _ _ _ _ _ _ _ _ _ _ w1194 w1249 _ _ w1326 w1362 _ w1483]
      tunnel: [w380 _ _ _ _ _ _ _ _ _ _ _ w1193 w1248 _ _ w1329 w1361 _ w1482] -> w336
      tunnel: [w379 _ _ _ _ _ _ _ _ _ _ _ w1192 w1247 _ _ w1328 w1360 _ w1481] -> w335
      tunnel: w334 -> [w349 _ _ _ _ _ _ _ _ _ _ _ _ _ _ _ w1325 w1357 _ w1480]
      tunnel: w333 -> [w352 _ _ _ _ _ _ _ _ _ _ _ _ _ _ _ w1324 w1356 _ w1479]
      tunnel: [w351 _ _ _ _ _ _ _ _ _ _ _ _ _ _ _ w1323 w1355 _ _] -> w332
      tunnel: [w350 _ _ _ _ _ _ _ _ _ _ _ _ _ _ _ w1322 w1354 _ _] -> w331
      tunnel: w330 -> [w348 _ _ _ _ _ _ _ _ _ _ _ _ _ _ _ w1321 _ _ _]
      tunnel: w329 -> [w347 _ _ _ _ _ _ _ _ _ _ _ _ _ _ _ w1320 _ _ _]
      tunnel: [w346 _ _ _ _ _ _ _ _ _ _ _ _ _ _ _ w1319 _ _ _] -> w328
      tunnel: [w345 _ _ _ _ _ _ _ _ _ _ _ _ _ _ _ w1318 _ _ _] -> w327
      event #0 {
        n145 = event-data() -> ()  [unwired: 1 in, 2 out]
        n146 = flat-sequence {
          tunnel: [w596] -> w378
          tunnel: [w572] -> w377
          tunnel: [w585] -> w376
          tunnel: [w563] -> w375
          tunnel: w349 -> [w562]
          tunnel: w352 -> [w561]
          tunnel: w378 -> [w602]
          tunnel: [w602] -> w374
          tunnel: w377 -> [w601]
          tunnel: [w601] -> w373
          tunnel: w376 -> [w600]
          tunnel: [w600] -> w372
          tunnel: w375 -> [w597]
          tunnel: [w597] -> w371
          tunnel: w374 -> [w609]
          tunnel: [w610] -> w370
          tunnel: w373 -> [w612]
          tunnel: [w611] -> w369
          tunnel: w372 -> [w608]
          tunnel: [w607] -> w368
          tunnel: w371 -> [w607]
          tunnel: w370 -> [w622]
          tunnel: w369 -> [w623]
          tunnel: [w621] -> w367
          tunnel: w368 -> [w625]
          tunnel: [w620] -> w366
          tunnel: [w708] -> w350
          tunnel: w367 -> [w708]
          tunnel: w366 -> [w688]
          tunnel: [w688] -> w351
          frame #0 {
            w567 = 0.1 ("Delay Time (s)")
            n147 = property on="Z Step SP" class="DigNum (strict)"() -> ("Maximum"=w587:dbl)  [unwired: 2 in, 2 out]
            n148 = property on="Z Step SP" class="DigNum (strict)"() -> ("Minimum"=w589:dbl)  [unwired: 2 in, 2 out]
            n149 = property on="Z steps/rev" class="DigNum (strict)"() -> ("Value"=w583:u32)  [unwired: 2 in, 2 out]
            n150 = property on="Z offset mm" class="DigNum (strict)"() -> ("Value"=w579:dbl)  [unwired: 2 in, 2 out]
            n151 = call "mDrive Send Command.vi"("error in (no error)"=w561, "Extra"="P", "Command"=T2."Print Parameter", "VISA resource name"=w562) -> ("error out"=w591:errorcluster, "read buffer"=w595:string, "VISA resource name out"=w593:refnum<visa-resource-name>)  [unwired: 3 in]
            n152 = call "Time Delay17"("error in (no error)"=w591, "Delay Time (s)"=w567) -> ("error out"=w590:errorcluster)  [unwired: 9 in]
            n153 = Decimal String To Number(string=w595, offset=0) -> (number=w575:i32)  [unwired: 1 in, 1 out]
            n154 = To Long Integer(number=w575) -> (32bit integer=w577:i32)
            n155 = property on="Z Step PV" class="DigNum (strict)"("Val(Sgnl)"=w577) -> ()  [unwired: 2 in, 2 out]
            n156 = To Long Integer(number=w587) -> (32bit integer=w586:i32)
            n157 = To Long Integer(number=w589) -> (32bit integer=w588:i32)
            n158 = call "mDrive Send Command.vi"("error in (no error)"=w590, "Extra"="MV", "Command"=T2."Print Parameter", "VISA resource name"=w593) -> ("error out"=w592:errorcluster, "read buffer"=w573:string, "VISA resource name out"=w596:refnum<visa-resource-name>)  [unwired: 3 in]
            n159 = call "Time Delay16"("error in (no error)"=w592, "Delay Time (s)"=w567) -> ("error out"=w572:errorcluster)  [unwired: 9 in]
            n160 = In Range and Coerce(upper limit=w586, x=w577, lower limit=w588) -> (In Range?=w585:bool)  [unwired: 1 out]
            n161 = To Double Precision Float(number=w577) -> (double precision float=w578:dbl)
            n162 = To Double Precision Float(number=w583) -> (double precision float=w584:dbl)
            n163 = Decimal String To Number(string=w573, offset=0 ("offset (0)")) -> (number=w566:i32)  [unwired: 1 in, 1 out]
            n164 = property on="Z in Range" class="Bool (strict)"("Val(Sgnl)"=w585) -> ()  [unwired: 2 in, 2 out]
            n165 = Divide(x=w578, y=w584) -> (x/y=w582:dbl)
            n166 = Number To Boolean Array(number=w566) -> (Boolean array=w565:bool[])
            n167 = property on="Z mm/rev" class="DigNum (strict)"() -> ("Value"=w581:dbl)  [unwired: 2 in, 2 out]
            n168 = Index Array(array=w565, index=0) -> (element=w563:bool)
            n169 = property on="Z in Motion" class="Bool (strict)"("Val(Sgnl)"=w563) -> ()  [unwired: 2 in, 2 out]
            n170 = Multiply(x=w582, y=w581) -> (x*y=w580:dbl)
            n171 = Add(x=w580, y=w579) -> (x+y=w576:dbl)
            n172 = property on="Z Position mm PV" class="DigNum (strict)"("Val(Sgnl)"=w576) -> ()  [unwired: 2 in, 2 out]
          }
          frame #1 {
            n173 = property on="Z Scan" class="Bool (strict)"() -> ("Value"=w598:bool)  [unwired: 2 in, 2 out]
            n174 = Or(x=w597, y=w598) -> (x .or. y?=w599:bool)
            n175 = case shown="True" w599 {
              frame #0 {
                n176 = property on="Z Go" class="Bool"("DisabledEnum"=T1."Enabled" ("Disabled")) -> ()  [unwired: 2 in, 2 out]
                n177 = property on="Z Scan OK" class="Bool"("DisabledEnum"=T1."Enabled" ("Disabled")) -> ()  [unwired: 2 in, 2 out]
              }
              frame #1 {
                n178 = property on="Z Go" class="Bool"("DisabledEnum"=T1."Disabled and Grayed Out" ("Disabled")) -> ()  [unwired: 2 in, 2 out]
                n179 = property on="Z Scan OK" class="Bool"("DisabledEnum"=T1."Disabled and Grayed Out" ("Disabled")) -> ()  [unwired: 2 in, 2 out]
              }
            }
          }
          frame #2 {
            n180 = case shown="False" w608 {
              tunnel: w609 -> [w615 w619]
              tunnel: [w616 w619] -> w610
              tunnel: [w617 w618] -> w611
              tunnel: w612 -> [w614 w618]
              frame #0 {
                n181 = call "mDrive Send Command.vi"("error in (no error)"=w614, "Command"=T2."Stop", "VISA resource name"=w615) -> ("error out"=w617:errorcluster, "VISA resource name out"=w616:refnum<visa-resource-name>)  [unwired: 4 in, 1 out]
              }
              frame #1 {
              }
            }
          }
          frame #3 {
            n182 = property on="Z Backlash corr" class="Bool (strict)"() -> ("Value"=w626:bool)  [unwired: 2 in, 2 out]
            n183 = Implies(1:w625, 2:w626) -> (0:w624:bool)
            n184 = case shown="False" w624 {
              tunnel: w623 -> [w633 w686]
              tunnel: w622 -> [w632 w687]
              tunnel: [w631 w686] -> w621
              tunnel: [w630 w687] -> w620
              frame #0 {
                # "Backlash"
                n185 = flat-sequence {
                  tunnel: [w648] -> w645
                  tunnel: [w650] -> w644
                  tunnel: [w649] -> w643
                  tunnel: w633 -> [w647]
                  tunnel: w632 -> [w646]
                  tunnel: w645 -> [w658]
                  tunnel: [w658] -> w642
                  tunnel: w644 -> [w657]
                  tunnel: w643 -> [w656]
                  tunnel: [w655] -> w641
                  tunnel: [w654] -> w640
                  tunnel: [w653] -> w629
                  tunnel: w642 -> [w668]
                  tunnel: w641 -> [w667]
                  tunnel: w640 -> [w665]
                  tunnel: [w666] -> w639
                  tunnel: [w665] -> w638
                  tunnel: [w664] -> w635
                  tunnel: [w663] -> w634
                  tunnel: w629 -> [w663]
                  tunnel: w639 -> [w679]
                  tunnel: w638 -> [w672]
                  tunnel: [w679] -> w637
                  tunnel: [w678] -> w636
                  tunnel: w635 -> [w678]
                  tunnel: w634 -> [w674]
                  tunnel: [w673] -> w627
                  tunnel: w637 -> [w683]
                  tunnel: w636 -> [w682]
                  tunnel: [w681] -> w631
                  tunnel: [w680] -> w628
                  tunnel: w627 -> [w680]
                  tunnel: [w685] -> w630
                  tunnel: w628 -> [w685]
                  frame #0 {
                    n186 = property on="Z Backlash steps/sec" class="DigNum (strict)"() -> ("Value"=w648:i32)  [unwired: 2 in, 2 out]
                    n187 = Number To Decimal String(number=w648) -> (decimal integer string=w651:string)  [unwired: 1 in]
                    n188 = call "mDrive Send Command.vi"("error in (no error)"=w647, "Extra"=w651, "Command"=T2."Max Velocity", "VISA resource name"=w646) -> ("error out"=w649:errorcluster, "VISA resource name out"=w650:refnum<visa-resource-name>)  [unwired: 3 in, 1 out]
                  }
                  frame #1 {
                    n189 = property on="Z Backlash" class="DigNum (strict)"() -> ("Value"=w653:i32)  [unwired: 2 in, 2 out]
                    n190 = Number To Decimal String(number=w653) -> (decimal integer string=w659:string)  [unwired: 1 in]
                    n191 = call "mDrive Send Command.vi"("error in (no error)"=w656, "Extra"=w659, "Command"=T2."Move to Relative Position", "VISA resource name"=w657) -> ("error out"=w655:errorcluster, "VISA resource name out"=w654:refnum<visa-resource-name>)  [unwired: 3 in, 1 out]
                  }
                  frame #2 {
                    n192 = To Double Precision Float(number=w663) -> (double precision float=w661:dbl)
                    n193 = To Double Precision Float(number=w668) -> (double precision float=w670:dbl)
                    n194 = Absolute Value(x=w661) -> (abs(x)=w662:dbl)
                    n195 = Divide(x=w662, y=w670) -> (x/y=w671:dbl)
                    n196 = Add(x=w671, y=0.3) -> (x+y=w664:dbl)
                    n197 = call "Time Delay18"("error in (no error)"=w667, "Delay Time (s)"=w664) -> ("error out"=w666:errorcluster)  [unwired: 9 in]
                  }
                  frame #3 {
                    n198 = Negate(x=w674) -> (-x=w675:i32)
                    n199 = Number To Decimal String(number=w675) -> (decimal integer string=w676:string)  [unwired: 1 in]
                    n200 = call "mDrive Send Command.vi"("Extra"=w676, "Command"=T2."Move to Relative Position", "VISA resource name"=w672) -> ("VISA resource name out"=w673:refnum<visa-resource-name>)  [unwired: 4 in, 2 out]
                  }
                  frame #4 {
                    n201 = call "Time Delay19"("error in (no error)"=w683, "Delay Time (s)"=w682) -> ("error out"=w681:errorcluster)  [unwired: 9 in]
                  }
                  frame #5 {
                    n202 = property on="Z Backlash corr" class="Bool (strict)"("Val(Sgnl)"=FALSE ("Value (Signaling)")) -> ()  [unwired: 2 in, 2 out]
                  }
                }
              }
              frame #1 {
              }
            }
          }
          frame #4 {
            n203 = property on="Z Step PV" class="DigNum (strict)"() -> ("Value"=w696:i32)  [unwired: 2 in, 2 out]
            n204 = property on="Z Step PV" class="DigNum (strict)"() -> ("Value"=w698:i32)  [unwired: 2 in, 2 out]
            n205 = property on="Z steps/rev" class="DigNum (strict)"() -> ("Value"=w700:u32)  [unwired: 2 in, 2 out]
            n206 = To Double Precision Float(number=w700) -> (double precision float=w694:dbl)
            n207 = property on="Z Step SP" class="DigNum (strict)"() -> ("Maximum"=w705:dbl)  [unwired: 2 in, 2 out]
            n208 = property on="Z Step SP" class="DigNum (strict)"() -> ("Minimum"=w706:dbl)  [unwired: 2 in, 2 out]
            n209 = To Double Precision Float(number=w696) -> (double precision float=w695:dbl)
            n210 = To Double Precision Float(number=w698) -> (double precision float=w697:dbl)
            n211 = Subtract(x=w706, y=w695) -> (x-y=w707:dbl)
            n212 = Subtract(x=w705, y=w697) -> (x-y=w704:dbl)
            n213 = property on="Z Velocity SP step/sec" class="DigNum (strict)"() -> ("Value"=w693:i32)  [unwired: 2 in, 2 out]
            n214 = property on="Z Scan Length SP steps" class="DigNum (strict)"() -> ("Value"=w702:i32)  [unwired: 2 in, 2 out]
            n215 = To Double Precision Float(number=w702) -> (double precision float=w701:dbl)
            n216 = To Double Precision Float(number=w693) -> (double precision float=w692:dbl)
            n217 = property on="Z Scan Length SP steps" class="DigNum (strict)"("Minimum"=w707) -> ()  [unwired: 2 in, 2 out]
            n218 = property on="Z Scan Length SP steps" class="DigNum (strict)"("Maximum"=w704) -> ()  [unwired: 2 in, 2 out]
            n219 = Divide(x=w701, y=w694) -> (x/y=w703:dbl)
            n220 = Divide(x=w692, y=w694) -> (x/y=w691:dbl)
            n221 = property on="Z mm/rev" class="DigNum (strict)"() -> ("Value"=w699:dbl)  [unwired: 2 in, 2 out]
            n222 = Multiply(x=w703, y=w699) -> (x*y=w690:dbl)
            n223 = Multiply(x=w699, y=w691) -> (x*y=w689:dbl)
            n224 = property on="Z Scan length MV mm" class="DigNum (strict)"("Value"=w690) -> ()  [unwired: 2 in, 2 out]
            n225 = property on="Z Scan velocity MV mm/sec" class="DigNum (strict)"("Val(Sgnl)"=w689) -> ()  [unwired: 2 in, 2 out]
          }
        }
        n226 = flat-sequence {
          tunnel: [w744] -> w395
          tunnel: [w720] -> w394
          tunnel: [w733] -> w393
          tunnel: [w711] -> w392
          tunnel: w382 -> [w710]
          tunnel: w381 -> [w709]
          tunnel: w395 -> [w750]
          tunnel: [w750] -> w391
          tunnel: w394 -> [w749]
          tunnel: [w749] -> w390
          tunnel: w393 -> [w748]
          tunnel: [w748] -> w389
          tunnel: w392 -> [w745]
          tunnel: [w745] -> w388
          tunnel: w391 -> [w757]
          tunnel: [w758] -> w387
          tunnel: w390 -> [w760]
          tunnel: [w759] -> w386
          tunnel: w389 -> [w756]
          tunnel: [w755] -> w385
          tunnel: w388 -> [w755]
          tunnel: w387 -> [w770]
          tunnel: w386 -> [w771]
          tunnel: [w769] -> w384
          tunnel: w385 -> [w773]
          tunnel: [w768] -> w383
          tunnel: [w856] -> w379
          tunnel: w384 -> [w856]
          tunnel: w383 -> [w836]
          tunnel: [w836] -> w380
          frame #0 {
            w715 = 0.1 ("Delay Time (s)")
            n227 = property on="X Step SP" class="DigNum (strict)"() -> ("Maximum"=w735:dbl)  [unwired: 2 in, 2 out]
            n228 = property on="X Step SP" class="DigNum (strict)"() -> ("Minimum"=w737:dbl)  [unwired: 2 in, 2 out]
            n229 = property on="X steps/rev" class="DigNum (strict)"() -> ("Value"=w731:u32)  [unwired: 2 in, 2 out]
            n230 = property on="X offset mm" class="DigNum (strict)"() -> ("Value"=w727:dbl)  [unwired: 2 in, 2 out]
            n231 = call "mDrive Send Command.vi"("error in (no error)"=w709, "Extra"="P", "Command"=T2."Print Parameter", "VISA resource name"=w710) -> ("error out"=w739:errorcluster, "read buffer"=w743:string, "VISA resource name out"=w741:refnum<visa-resource-name>)  [unwired: 3 in]
            n232 = call "Time Delay12"("error in (no error)"=w739, "Delay Time (s)"=w715) -> ("error out"=w738:errorcluster)  [unwired: 9 in]
            n233 = Decimal String To Number(string=w743, offset=0) -> (number=w723:i32)  [unwired: 1 in, 1 out]
            n234 = To Long Integer(number=w723) -> (32bit integer=w725:i32)
            n235 = property on="X Step PV" class="DigNum (strict)"("Val(Sgnl)"=w725) -> ()  [unwired: 2 in, 2 out]
            n236 = To Long Integer(number=w735) -> (32bit integer=w734:i32)
            n237 = To Long Integer(number=w737) -> (32bit integer=w736:i32)
            n238 = call "mDrive Send Command.vi"("error in (no error)"=w738, "Extra"="MV", "Command"=T2."Print Parameter", "VISA resource name"=w741) -> ("error out"=w740:errorcluster, "read buffer"=w721:string, "VISA resource name out"=w744:refnum<visa-resource-name>)  [unwired: 3 in]
            n239 = call "Time Delay11"("error in (no error)"=w740, "Delay Time (s)"=w715) -> ("error out"=w720:errorcluster)  [unwired: 9 in]
            n240 = In Range and Coerce(upper limit=w734, x=w725, lower limit=w736) -> (In Range?=w733:bool)  [unwired: 1 out]
            n241 = To Double Precision Float(number=w725) -> (double precision float=w726:dbl)
            n242 = To Double Precision Float(number=w731) -> (double precision float=w732:dbl)
            n243 = Decimal String To Number(string=w721, offset=0 ("offset (0)")) -> (number=w714:i32)  [unwired: 1 in, 1 out]
            n244 = property on="X  in Range" class="Bool (strict)"("Val(Sgnl)"=w733) -> ()  [unwired: 2 in, 2 out]
            n245 = Divide(x=w726, y=w732) -> (x/y=w730:dbl)
            n246 = Number To Boolean Array(number=w714) -> (Boolean array=w713:bool[])
            n247 = property on="X mm/rev" class="DigNum (strict)"() -> ("Value"=w729:dbl)  [unwired: 2 in, 2 out]
            n248 = Index Array(array=w713, index=0) -> (element=w711:bool)
            n249 = property on="X  in Motion" class="Bool (strict)"("Val(Sgnl)"=w711) -> ()  [unwired: 2 in, 2 out]
            n250 = Multiply(x=w730, y=w729) -> (x*y=w728:dbl)
            n251 = Add(x=w728, y=w727) -> (x+y=w724:dbl)
            n252 = property on="X Position mm PV" class="DigNum (strict)"("Val(Sgnl)"=w724) -> ()  [unwired: 2 in, 2 out]
          }
          frame #1 {
            n253 = property on="X Scan" class="Bool (strict)"() -> ("Value"=w746:bool)  [unwired: 2 in, 2 out]
            n254 = Or(x=w745, y=w746) -> (x .or. y?=w747:bool)
            n255 = case shown="False" w747 {
              frame #0 {
                n256 = property on="X Go" class="Bool"("DisabledEnum"=T1."Enabled" ("Disabled")) -> ()  [unwired: 2 in, 2 out]
                n257 = property on="X Scan OK" class="Bool"("DisabledEnum"=T1."Enabled" ("Disabled")) -> ()  [unwired: 2 in, 2 out]
              }
              frame #1 {
                n258 = property on="X Go" class="Bool"("DisabledEnum"=T1."Disabled and Grayed Out" ("Disabled")) -> ()  [unwired: 2 in, 2 out]
                n259 = property on="X Scan set" class="Bool"("DisabledEnum"=T1."Disabled and Grayed Out" ("Disabled")) -> ()  [unwired: 2 in, 2 out]
              }
            }
          }
          frame #2 {
            n260 = case shown="False" w756 {
              tunnel: w757 -> [w763 w767]
              tunnel: [w764 w767] -> w758
              tunnel: [w765 w766] -> w759
              tunnel: w760 -> [w762 w766]
              frame #0 {
                n261 = call "mDrive Send Command.vi"("error in (no error)"=w762, "Command"=T2."Stop", "VISA resource name"=w763) -> ("error out"=w765:errorcluster, "VISA resource name out"=w764:refnum<visa-resource-name>)  [unwired: 4 in, 1 out]
              }
              frame #1 {
              }
            }
          }
          frame #3 {
            n262 = property on="X Backlash corr" class="Bool (strict)"() -> ("Value"=w774:bool)  [unwired: 2 in, 2 out]
            n263 = Implies(1:w773, 2:w774) -> (0:w772:bool)
            n264 = case shown="False" w772 {
              tunnel: w771 -> [w781 w834]
              tunnel: w770 -> [w780 w835]
              tunnel: [w779 w834] -> w769
              tunnel: [w778 w835] -> w768
              frame #0 {
                # "Backlash"
                n265 = flat-sequence {
                  tunnel: [w796] -> w793
                  tunnel: [w798] -> w792
                  tunnel: [w797] -> w791
                  tunnel: w781 -> [w795]
                  tunnel: w780 -> [w794]
                  tunnel: w793 -> [w806]
                  tunnel: [w806] -> w790
                  tunnel: w792 -> [w805]
                  tunnel: w791 -> [w804]
                  tunnel: [w803] -> w789
                  tunnel: [w802] -> w788
                  tunnel: [w801] -> w777
                  tunnel: w790 -> [w816]
                  tunnel: w789 -> [w815]
                  tunnel: w788 -> [w813]
                  tunnel: [w814] -> w787
                  tunnel: [w813] -> w786
                  tunnel: [w812] -> w783
                  tunnel: [w811] -> w782
                  tunnel: w777 -> [w811]
                  tunnel: w787 -> [w827]
                  tunnel: w786 -> [w820]
                  tunnel: [w827] -> w785
                  tunnel: [w826] -> w784
                  tunnel: w783 -> [w826]
                  tunnel: w782 -> [w822]
                  tunnel: [w821] -> w775
                  tunnel: w785 -> [w831]
                  tunnel: w784 -> [w830]
                  tunnel: [w829] -> w779
                  tunnel: [w828] -> w776
                  tunnel: w775 -> [w828]
                  tunnel: [w833] -> w778
                  tunnel: w776 -> [w833]
                  frame #0 {
                    n266 = property on="X Backlash steps/sec" class="DigNum (strict)"() -> ("Value"=w796:i32)  [unwired: 2 in, 2 out]
                    n267 = Number To Decimal String(number=w796) -> (decimal integer string=w799:string)  [unwired: 1 in]
                    n268 = call "mDrive Send Command.vi"("error in (no error)"=w795, "Extra"=w799, "Command"=T2."Max Velocity", "VISA resource name"=w794) -> ("error out"=w797:errorcluster, "VISA resource name out"=w798:refnum<visa-resource-name>)  [unwired: 3 in, 1 out]
                  }
                  frame #1 {
                    n269 = property on="X Backlash" class="DigNum (strict)"() -> ("Value"=w801:i32)  [unwired: 2 in, 2 out]
                    n270 = Number To Decimal String(number=w801) -> (decimal integer string=w807:string)  [unwired: 1 in]
                    n271 = call "mDrive Send Command.vi"("error in (no error)"=w804, "Extra"=w807, "Command"=T2."Move to Relative Position", "VISA resource name"=w805) -> ("error out"=w803:errorcluster, "VISA resource name out"=w802:refnum<visa-resource-name>)  [unwired: 3 in, 1 out]
                  }
                  frame #2 {
                    n272 = To Double Precision Float(number=w811) -> (double precision float=w809:dbl)
                    n273 = To Double Precision Float(number=w816) -> (double precision float=w818:dbl)
                    n274 = Absolute Value(x=w809) -> (abs(x)=w810:dbl)
                    n275 = Divide(x=w810, y=w818) -> (x/y=w819:dbl)
                    n276 = Add(x=w819, y=0.3) -> (x+y=w812:dbl)
                    n277 = call "Time Delay13"("error in (no error)"=w815, "Delay Time (s)"=w812) -> ("error out"=w814:errorcluster)  [unwired: 9 in]
                  }
                  frame #3 {
                    n278 = Negate(x=w822) -> (-x=w823:i32)
                    n279 = Number To Decimal String(number=w823) -> (decimal integer string=w824:string)  [unwired: 1 in]
                    n280 = call "mDrive Send Command.vi"("Extra"=w824, "Command"=T2."Move to Relative Position", "VISA resource name"=w820) -> ("VISA resource name out"=w821:refnum<visa-resource-name>)  [unwired: 4 in, 2 out]
                  }
                  frame #4 {
                    n281 = call "Time Delay14"("error in (no error)"=w831, "Delay Time (s)"=w830) -> ("error out"=w829:errorcluster)  [unwired: 9 in]
                  }
                  frame #5 {
                    n282 = property on="X Backlash corr" class="Bool (strict)"("Val(Sgnl)"=FALSE ("Value (Signaling)")) -> ()  [unwired: 2 in, 2 out]
                  }
                }
              }
              frame #1 {
              }
            }
          }
          frame #4 {
            n283 = property on="X Step PV" class="DigNum (strict)"() -> ("Value"=w846:i32)  [unwired: 2 in, 2 out]
            n284 = property on="X Step PV" class="DigNum (strict)"() -> ("Value"=w844:i32)  [unwired: 2 in, 2 out]
            n285 = property on="X steps/rev" class="DigNum (strict)"() -> ("Value"=w848:u32)  [unwired: 2 in, 2 out]
            n286 = To Double Precision Float(number=w848) -> (double precision float=w842:dbl)
            n287 = property on="X Step SP" class="DigNum (strict)"() -> ("Maximum"=w853:dbl)  [unwired: 2 in, 2 out]
            n288 = property on="X Step SP" class="DigNum (strict)"() -> ("Minimum"=w854:dbl)  [unwired: 2 in, 2 out]
            n289 = To Double Precision Float(number=w844) -> (double precision float=w843:dbl)
            n290 = To Double Precision Float(number=w846) -> (double precision float=w845:dbl)
            n291 = Subtract(x=w853, y=w845) -> (x-y=w852:dbl)
            n292 = Subtract(x=w854, y=w843) -> (x-y=w855:dbl)
            n293 = property on="X Scan Length SP steps" class="DigNum (strict)"() -> ("Value"=w841:i32)  [unwired: 2 in, 2 out]
            n294 = property on="X Scan Velocity SP steps/sec" class="DigNum (strict)"() -> ("Value"=w850:i32)  [unwired: 2 in, 2 out]
            n295 = To Double Precision Float(number=w841) -> (double precision float=w840:dbl)
            n296 = property on="X Scan Length SP steps" class="DigNum (strict)"("Maximum"=w852) -> ()  [unwired: 2 in, 2 out]
            n297 = property on="X Scan Length SP steps" class="DigNum (strict)"("Minimum"=w855) -> ()  [unwired: 2 in, 2 out]
            n298 = Divide(x=w840, y=w842) -> (x/y=w839:dbl)
            n299 = To Double Precision Float(number=w850) -> (double precision float=w849:dbl)
            n300 = property on="X mm/rev" class="DigNum (strict)"() -> ("Value"=w847:dbl)  [unwired: 2 in, 2 out]
            n301 = Divide(x=w849, y=w842) -> (x/y=w851:dbl)
            n302 = Multiply(x=w847, y=w839) -> (x*y=w837:dbl)
            n303 = Multiply(x=w851, y=w847) -> (x*y=w838:dbl)
            n304 = property on="X Scan length MV mm" class="DigNum (strict)"("Val(Sgnl)"=w837) -> ()  [unwired: 2 in, 2 out]
            n305 = property on="X Scan velocity MV mm/sec" class="DigNum (strict)"("Value"=w838) -> ()  [unwired: 2 in, 2 out]
          }
        }
        n306 = flat-sequence {
          tunnel: w412 -> [w887]
          tunnel: w409 -> [w886]
          tunnel: [w892] -> w408
          tunnel: [w866] -> w406
          tunnel: [w879] -> w404
          tunnel: [w857] -> w402
          tunnel: w408 -> [w898]
          tunnel: [w898] -> w407
          tunnel: w406 -> [w897]
          tunnel: [w897] -> w405
          tunnel: w404 -> [w896]
          tunnel: [w896] -> w403
          tunnel: w402 -> [w893]
          tunnel: [w893] -> w397
          tunnel: w407 -> [w905]
          tunnel: [w906] -> w401
          tunnel: w405 -> [w908]
          tunnel: [w907] -> w400
          tunnel: w403 -> [w904]
          tunnel: [w903] -> w398
          tunnel: w397 -> [w903]
          tunnel: w401 -> [w918]
          tunnel: w400 -> [w919]
          tunnel: [w917] -> w399
          tunnel: w398 -> [w921]
          tunnel: [w916] -> w396
          tunnel: [w1003] -> w411
          tunnel: [w1004] -> w410
          tunnel: w399 -> [w1003]
          tunnel: w396 -> [w1004]
          frame #0 {
            w861 = 0.1 ("Delay Time (s)")
            n307 = property on="Y Step SP" class="DigNum (strict)"() -> ("Maximum"=w881:dbl)  [unwired: 2 in, 2 out]
            n308 = property on="Y Step SP" class="DigNum (strict)"() -> ("Minimum"=w883:dbl)  [unwired: 2 in, 2 out]
            n309 = property on="Y steps/rev" class="DigNum (strict)"() -> ("Value"=w877:u32)  [unwired: 2 in, 2 out]
            n310 = property on="Y offset mm" class="DigNum (strict)"() -> ("Value"=w873:dbl)  [unwired: 2 in, 2 out]
            n311 = call "mDrive Send Command.vi"("error in (no error)"=w887, "Extra"="P", "Command"=T2."Print Parameter", "VISA resource name"=w886) -> ("error out"=w885:errorcluster, "read buffer"=w891:string, "VISA resource name out"=w889:refnum<visa-resource-name>)  [unwired: 3 in]
            n312 = call "Time Delay4"("error in (no error)"=w885, "Delay Time (s)"=w861) -> ("error out"=w884:errorcluster)  [unwired: 9 in]
            n313 = Decimal String To Number(string=w891, offset=0) -> (number=w869:i32)  [unwired: 1 in, 1 out]
            n314 = To Long Integer(number=w869) -> (32bit integer=w871:i32)
            n315 = property on="Y Step PV" class="DigNum (strict)"("Val(Sgnl)"=w871) -> ()  [unwired: 2 in, 2 out]
            n316 = To Long Integer(number=w881) -> (32bit integer=w880:i32)
            n317 = To Long Integer(number=w883) -> (32bit integer=w882:i32)
            n318 = call "mDrive Send Command.vi"("error in (no error)"=w884, "Extra"="MV", "Command"=T2."Print Parameter", "VISA resource name"=w889) -> ("error out"=w888:errorcluster, "read buffer"=w867:string, "VISA resource name out"=w892:refnum<visa-resource-name>)  [unwired: 3 in]
            n319 = call "Time Delay3"("error in (no error)"=w888, "Delay Time (s)"=w861) -> ("error out"=w866:errorcluster)  [unwired: 9 in]
            n320 = In Range and Coerce(upper limit=w880, x=w871, lower limit=w882) -> (In Range?=w879:bool)  [unwired: 1 out]
            n321 = To Double Precision Float(number=w871) -> (double precision float=w872:dbl)
            n322 = To Double Precision Float(number=w877) -> (double precision float=w878:dbl)
            n323 = Decimal String To Number(string=w867, offset=0 ("offset (0)")) -> (number=w860:i32)  [unwired: 1 in, 1 out]
            n324 = property on="Y in Range" class="Bool (strict)"("Val(Sgnl)"=w879) -> ()  [unwired: 2 in, 2 out]
            n325 = Divide(x=w872, y=w878) -> (x/y=w876:dbl)
            n326 = Number To Boolean Array(number=w860) -> (Boolean array=w859:bool[])
            n327 = property on="Y mm/rev" class="DigNum (strict)"() -> ("Value"=w875:dbl)  [unwired: 2 in, 2 out]
            n328 = Index Array(array=w859, index=0) -> (element=w857:bool)
            n329 = property on="Y in Motion" class="Bool (strict)"("Val(Sgnl)"=w857) -> ()  [unwired: 2 in, 2 out]
            n330 = Multiply(x=w876, y=w875) -> (x*y=w874:dbl)
            n331 = Add(x=w874, y=w873) -> (x+y=w870:dbl)
            n332 = property on="Y Position mm PV" class="DigNum (strict)"("Val(Sgnl)"=w870) -> ()  [unwired: 2 in, 2 out]
          }
          frame #1 {
            n333 = property on="Y Scan" class="Bool (strict)"() -> ("Value"=w894:bool)  [unwired: 2 in, 2 out]
            n334 = Or(x=w893, y=w894) -> (x .or. y?=w895:bool)
            n335 = case shown="True" w895 {
              frame #0 {
                n336 = property on="Y Go" class="Bool"("DisabledEnum"=T1."Enabled" ("Disabled")) -> ()  [unwired: 2 in, 2 out]
                n337 = property on="Y Scan OK" class="Bool"("DisabledEnum"=T1."Enabled" ("Disabled")) -> ()  [unwired: 2 in, 2 out]
              }
              frame #1 {
                n338 = property on="Y Go" class="Bool"("DisabledEnum"=T1."Disabled and Grayed Out" ("Disabled")) -> ()  [unwired: 2 in, 2 out]
                n339 = property on="Y Scan OK" class="Bool"("DisabledEnum"=T1."Disabled and Grayed Out" ("Disabled")) -> ()  [unwired: 2 in, 2 out]
              }
            }
          }
          frame #2 {
            n340 = case shown="False" w904 {
              tunnel: w905 -> [w911 w915]
              tunnel: [w912 w915] -> w906
              tunnel: [w913 w914] -> w907
              tunnel: w908 -> [w910 w914]
              frame #0 {
                n341 = call "mDrive Send Command.vi"("error in (no error)"=w910, "Command"=T2."Stop", "VISA resource name"=w911) -> ("error out"=w913:errorcluster, "VISA resource name out"=w912:refnum<visa-resource-name>)  [unwired: 4 in, 1 out]
              }
              frame #1 {
              }
            }
          }
          frame #3 {
            n342 = property on="Y Backlash corr" class="Bool (strict)"() -> ("Value"=w922:bool)  [unwired: 2 in, 2 out]
            n343 = Implies(1:w921, 2:w922) -> (0:w920:bool)
            n344 = case shown="False" w920 {
              tunnel: w919 -> [w929 w982]
              tunnel: w918 -> [w928 w983]
              tunnel: [w927 w982] -> w917
              tunnel: [w926 w983] -> w916
              frame #0 {
                # "Backlash"
                n345 = flat-sequence {
                  tunnel: [w944] -> w941
                  tunnel: [w946] -> w940
                  tunnel: [w945] -> w939
                  tunnel: w929 -> [w943]
                  tunnel: w928 -> [w942]
                  tunnel: w941 -> [w954]
                  tunnel: [w954] -> w938
                  tunnel: w940 -> [w953]
                  tunnel: w939 -> [w952]
                  tunnel: [w951] -> w937
                  tunnel: [w950] -> w936
                  tunnel: [w949] -> w925
                  tunnel: w938 -> [w964]
                  tunnel: w937 -> [w963]
                  tunnel: w936 -> [w961]
                  tunnel: [w962] -> w935
                  tunnel: [w961] -> w934
                  tunnel: [w960] -> w931
                  tunnel: [w959] -> w930
                  tunnel: w925 -> [w959]
                  tunnel: w935 -> [w975]
                  tunnel: w934 -> [w968]
                  tunnel: [w975] -> w933
                  tunnel: [w974] -> w932
                  tunnel: w931 -> [w974]
                  tunnel: w930 -> [w970]
                  tunnel: [w969] -> w923
                  tunnel: w933 -> [w979]
                  tunnel: w932 -> [w978]
                  tunnel: [w977] -> w927
                  tunnel: [w976] -> w924
                  tunnel: w923 -> [w976]
                  tunnel: [w981] -> w926
                  tunnel: w924 -> [w981]
                  frame #0 {
                    n346 = property on="Y Backlash steps/sec" class="DigNum (strict)"() -> ("Value"=w944:i32)  [unwired: 2 in, 2 out]
                    n347 = Number To Decimal String(number=w944) -> (decimal integer string=w947:string)  [unwired: 1 in]
                    n348 = call "mDrive Send Command.vi"("error in (no error)"=w943, "Extra"=w947, "Command"=T2."Max Velocity", "VISA resource name"=w942) -> ("error out"=w945:errorcluster, "VISA resource name out"=w946:refnum<visa-resource-name>)  [unwired: 3 in, 1 out]
                  }
                  frame #1 {
                    n349 = property on="Y Backlash" class="DigNum (strict)"() -> ("Value"=w949:i32)  [unwired: 2 in, 2 out]
                    n350 = Number To Decimal String(number=w949) -> (decimal integer string=w955:string)  [unwired: 1 in]
                    n351 = call "mDrive Send Command.vi"("error in (no error)"=w952, "Extra"=w955, "Command"=T2."Move to Relative Position", "VISA resource name"=w953) -> ("error out"=w951:errorcluster, "VISA resource name out"=w950:refnum<visa-resource-name>)  [unwired: 3 in, 1 out]
                  }
                  frame #2 {
                    n352 = To Double Precision Float(number=w959) -> (double precision float=w957:dbl)
                    n353 = To Double Precision Float(number=w964) -> (double precision float=w966:dbl)
                    n354 = Absolute Value(x=w957) -> (abs(x)=w958:dbl)
                    n355 = Divide(x=w958, y=w966) -> (x/y=w967:dbl)
                    n356 = Add(x=w967, y=0.3) -> (x+y=w960:dbl)
                    n357 = call "Time Delay8"("error in (no error)"=w963, "Delay Time (s)"=w960) -> ("error out"=w962:errorcluster)  [unwired: 9 in]
                  }
                  frame #3 {
                    n358 = Negate(x=w970) -> (-x=w971:i32)
                    n359 = Number To Decimal String(number=w971) -> (decimal integer string=w972:string)  [unwired: 1 in]
                    n360 = call "mDrive Send Command.vi"("Extra"=w972, "Command"=T2."Move to Relative Position", "VISA resource name"=w968) -> ("VISA resource name out"=w969:refnum<visa-resource-name>)  [unwired: 4 in, 2 out]
                  }
                  frame #4 {
                    n361 = call "Time Delay2"("error in (no error)"=w979, "Delay Time (s)"=w978) -> ("error out"=w977:errorcluster)  [unwired: 9 in]
                  }
                  frame #5 {
                    n362 = property on="Y Backlash corr" class="Bool (strict)"("Val(Sgnl)"=FALSE ("Value (Signaling)")) -> ()  [unwired: 2 in, 2 out]
                  }
                }
              }
              frame #1 {
              }
            }
          }
          frame #4 {
            n363 = property on="Y Step PV" class="DigNum (strict)"() -> ("Value"=w993:i32)  [unwired: 2 in, 2 out]
            n364 = property on="Y Step PV" class="DigNum (strict)"() -> ("Value"=w991:i32)  [unwired: 2 in, 2 out]
            n365 = property on="Y steps/rev" class="DigNum (strict)"() -> ("Value"=w995:u32)  [unwired: 2 in, 2 out]
            n366 = To Double Precision Float(number=w995) -> (double precision float=w989:dbl)
            n367 = property on="Y Step SP" class="DigNum (strict)"() -> ("Maximum"=w1000:dbl)  [unwired: 2 in, 2 out]
            n368 = property on="Y Step SP" class="DigNum (strict)"() -> ("Minimum"=w1001:dbl)  [unwired: 2 in, 2 out]
            n369 = To Double Precision Float(number=w991) -> (double precision float=w990:dbl)
            n370 = To Double Precision Float(number=w993) -> (double precision float=w992:dbl)
            n371 = Subtract(x=w1000, y=w992) -> (x-y=w999:dbl)
            n372 = Subtract(x=w1001, y=w990) -> (x-y=w1002:dbl)
            n373 = property on="Y Scan Length SP steps" class="DigNum (strict)"() -> ("Value"=w997:i32)  [unwired: 2 in, 2 out]
            n374 = property on="Y Scan Velocity SP steps/sec" class="DigNum (strict)"() -> ("Value"=w988:i32)  [unwired: 2 in, 2 out]
            n375 = To Double Precision Float(number=w997) -> (double precision float=w996:dbl)
            n376 = property on="Y Scan Length SP steps" class="DigNum (strict)"("Maximum"=w999) -> ()  [unwired: 2 in, 2 out]
            n377 = property on="Y Scan Length SP steps" class="DigNum (strict)"("Minimum"=w1002) -> ()  [unwired: 2 in, 2 out]
            n378 = Divide(x=w996, y=w989) -> (x/y=w998:dbl)
            n379 = To Double Precision Float(number=w988) -> (double precision float=w987:dbl)
            n380 = property on="Y mm/rev" class="DigNum (strict)"() -> ("Value"=w994:dbl)  [unwired: 2 in, 2 out]
            n381 = Multiply(x=w998, y=w994) -> (x*y=w985:dbl)
            n382 = Divide(x=w987, y=w989) -> (x/y=w986:dbl)
            n383 = Multiply(x=w994, y=w986) -> (x*y=w984:dbl)
            n384 = property on="Y Scan length MV mm" class="DigNum (strict)"("Value"=w985) -> ()  [unwired: 2 in, 2 out]
            n385 = property on="Y Scan velocity MV mm/sec" class="DigNum (strict)"("Val(Sgnl)"=w984) -> ()  [unwired: 2 in, 2 out]
          }
        }
        n386 = flat-sequence {
          tunnel: [w448] -> w365
          tunnel: [w424] -> w364
          tunnel: [w437] -> w363
          tunnel: [w415] -> w362
          tunnel: w348 -> [w414]
          tunnel: w347 -> [w413]
          tunnel: w365 -> [w454]
          tunnel: [w454] -> w361
          tunnel: w364 -> [w453]
          tunnel: [w453] -> w360
          tunnel: w363 -> [w452]
          tunnel: [w452] -> w359
          tunnel: w362 -> [w449]
          tunnel: [w449] -> w358
          tunnel: w361 -> [w461]
          tunnel: [w462] -> w357
          tunnel: w360 -> [w464]
          tunnel: [w463] -> w356
          tunnel: w359 -> [w460]
          tunnel: [w459] -> w355
          tunnel: w358 -> [w459]
          tunnel: w357 -> [w474]
          tunnel: w356 -> [w475]
          tunnel: [w473] -> w354
          tunnel: w355 -> [w477]
          tunnel: [w472] -> w353
          tunnel: [w560] -> w345
          tunnel: w354 -> [w560]
          tunnel: w353 -> [w540]
          tunnel: [w540] -> w346
          frame #0 {
            w419 = 0.1 ("Delay Time (s)")
            n387 = property on="R Step SP" class="DigNum (strict)"() -> ("Maximum"=w439:dbl)  [unwired: 2 in, 2 out]
            n388 = property on="R Step SP" class="DigNum (strict)"() -> ("Minimum"=w441:dbl)  [unwired: 2 in, 2 out]
            n389 = property on="R steps/rev" class="DigNum (strict)"() -> ("Value"=w435:u32)  [unwired: 2 in, 2 out]
            n390 = property on="R offset deg" class="DigNum (strict)"() -> ("Value"=w431:dbl)  [unwired: 2 in, 2 out]
            n391 = call "mDrive Send Command.vi"("error in (no error)"=w413, "Extra"="P", "Command"=T2."Print Parameter", "VISA resource name"=w414) -> ("error out"=w443:errorcluster, "read buffer"=w447:string, "VISA resource name out"=w445:refnum<visa-resource-name>)  [unwired: 3 in]
            n392 = call "Time Delay21"("error in (no error)"=w443, "Delay Time (s)"=w419) -> ("error out"=w442:errorcluster)  [unwired: 9 in]
            n393 = Decimal String To Number(string=w447, offset=0) -> (number=w427:i32)  [unwired: 1 in, 1 out]
            n394 = To Long Integer(number=w427) -> (32bit integer=w429:i32)
            n395 = property on="R Step PV" class="DigNum (strict)"("Val(Sgnl)"=w429) -> ()  [unwired: 2 in, 2 out]
            n396 = To Long Integer(number=w439) -> (32bit integer=w438:i32)
            n397 = To Long Integer(number=w441) -> (32bit integer=w440:i32)
            n398 = call "mDrive Send Command.vi"("error in (no error)"=w442, "Extra"="MV", "Command"=T2."Print Parameter", "VISA resource name"=w445) -> ("error out"=w444:errorcluster, "read buffer"=w425:string, "VISA resource name out"=w448:refnum<visa-resource-name>)  [unwired: 3 in]
            n399 = call "Time Delay20"("error in (no error)"=w444, "Delay Time (s)"=w419) -> ("error out"=w424:errorcluster)  [unwired: 9 in]
            n400 = In Range and Coerce(upper limit=w438, x=w429, lower limit=w440) -> (In Range?=w437:bool)  [unwired: 1 out]
            n401 = To Double Precision Float(number=w429) -> (double precision float=w430:dbl)
            n402 = To Double Precision Float(number=w435) -> (double precision float=w436:dbl)
            n403 = Decimal String To Number(string=w425, offset=0 ("offset (0)")) -> (number=w418:i32)  [unwired: 1 in, 1 out]
            n404 = property on="R in Range" class="Bool (strict)"("Val(Sgnl)"=w437) -> ()  [unwired: 2 in, 2 out]
            n405 = Divide(x=w430, y=w436) -> (x/y=w434:dbl)
            n406 = Number To Boolean Array(number=w418) -> (Boolean array=w417:bool[])
            n407 = property on="R deg/rev" class="DigNum (strict)"() -> ("Value"=w433:dbl)  [unwired: 2 in, 2 out]
            n408 = Index Array(array=w417, index=0) -> (element=w415:bool)
            n409 = property on="R in Motion" class="Bool (strict)"("Val(Sgnl)"=w415) -> ()  [unwired: 2 in, 2 out]
            n410 = Multiply(x=w434, y=w433) -> (x*y=w432:dbl)
            n411 = Add(x=w432, y=w431) -> (x+y=w428:dbl)
            n412 = property on="R Position deg PV" class="DigNum (strict)"("Val(Sgnl)"=w428) -> ()  [unwired: 2 in, 2 out]
          }
          frame #1 {
            n413 = property on="R Scan" class="Bool (strict)"() -> ("Value"=w450:bool)  [unwired: 2 in, 2 out]
            n414 = Or(x=w449, y=w450) -> (x .or. y?=w451:bool)
            n415 = case shown="True" w451 {
              frame #0 {
                n416 = property on="R Go" class="Bool"("DisabledEnum"=T1."Enabled" ("Disabled")) -> ()  [unwired: 2 in, 2 out]
                n417 = property on="R Scan OK" class="Bool"("DisabledEnum"=T1."Enabled" ("Disabled")) -> ()  [unwired: 2 in, 2 out]
              }
              frame #1 {
                n418 = property on="R Go" class="Bool"("DisabledEnum"=T1."Disabled and Grayed Out" ("Disabled")) -> ()  [unwired: 2 in, 2 out]
                n419 = property on="R Scan OK" class="Bool"("DisabledEnum"=T1."Disabled and Grayed Out" ("Disabled")) -> ()  [unwired: 2 in, 2 out]
              }
            }
          }
          frame #2 {
            n420 = case shown="False" w460 {
              tunnel: w461 -> [w467 w471]
              tunnel: [w468 w471] -> w462
              tunnel: [w469 w470] -> w463
              tunnel: w464 -> [w466 w470]
              frame #0 {
                n421 = call "mDrive Send Command.vi"("error in (no error)"=w466, "Command"=T2."Stop", "VISA resource name"=w467) -> ("error out"=w469:errorcluster, "VISA resource name out"=w468:refnum<visa-resource-name>)  [unwired: 4 in, 1 out]
              }
              frame #1 {
              }
            }
          }
          frame #3 {
            n422 = property on="R Backlash corr" class="Bool (strict)"() -> ("Value"=w478:bool)  [unwired: 2 in, 2 out]
            n423 = Implies(1:w477, 2:w478) -> (0:w476:bool)
            n424 = case shown="False" w476 {
              tunnel: w475 -> [w485 w538]
              tunnel: w474 -> [w484 w539]
              tunnel: [w483 w538] -> w473
              tunnel: [w482 w539] -> w472
              frame #0 {
                # "Backlash"
                n425 = flat-sequence {
                  tunnel: [w500] -> w497
                  tunnel: [w502] -> w496
                  tunnel: [w501] -> w495
                  tunnel: w485 -> [w499]
                  tunnel: w484 -> [w498]
                  tunnel: w497 -> [w510]
                  tunnel: [w510] -> w494
                  tunnel: w496 -> [w509]
                  tunnel: w495 -> [w508]
                  tunnel: [w507] -> w493
                  tunnel: [w506] -> w492
                  tunnel: [w505] -> w481
                  tunnel: w494 -> [w520]
                  tunnel: w493 -> [w519]
                  tunnel: w492 -> [w517]
                  tunnel: [w518] -> w491
                  tunnel: [w517] -> w490
                  tunnel: [w516] -> w487
                  tunnel: [w515] -> w486
                  tunnel: w481 -> [w515]
                  tunnel: w491 -> [w531]
                  tunnel: w490 -> [w524]
                  tunnel: [w531] -> w489
                  tunnel: [w530] -> w488
                  tunnel: w487 -> [w530]
                  tunnel: w486 -> [w526]
                  tunnel: [w525] -> w479
                  tunnel: w489 -> [w535]
                  tunnel: w488 -> [w534]
                  tunnel: [w533] -> w483
                  tunnel: [w532] -> w480
                  tunnel: w479 -> [w532]
                  tunnel: [w537] -> w482
                  tunnel: w480 -> [w537]
                  frame #0 {
                    n426 = property on="R Backlash steps/sec" class="DigNum (strict)"() -> ("Value"=w500:i32)  [unwired: 2 in, 2 out]
                    n427 = Number To Decimal String(number=w500) -> (decimal integer string=w503:string)  [unwired: 1 in]
                    n428 = call "mDrive Send Command.vi"("error in (no error)"=w499, "Extra"=w503, "Command"=T2."Max Velocity", "VISA resource name"=w498) -> ("error out"=w501:errorcluster, "VISA resource name out"=w502:refnum<visa-resource-name>)  [unwired: 3 in, 1 out]
                  }
                  frame #1 {
                    n429 = property on="R Backlash" class="DigNum (strict)"() -> ("Value"=w505:i32)  [unwired: 2 in, 2 out]
                    n430 = Number To Decimal String(number=w505) -> (decimal integer string=w511:string)  [unwired: 1 in]
                    n431 = call "mDrive Send Command.vi"("error in (no error)"=w508, "Extra"=w511, "Command"=T2."Move to Relative Position", "VISA resource name"=w509) -> ("error out"=w507:errorcluster, "VISA resource name out"=w506:refnum<visa-resource-name>)  [unwired: 3 in, 1 out]
                  }
                  frame #2 {
                    n432 = To Double Precision Float(number=w515) -> (double precision float=w513:dbl)
                    n433 = To Double Precision Float(number=w520) -> (double precision float=w522:dbl)
                    n434 = Absolute Value(x=w513) -> (abs(x)=w514:dbl)
                    n435 = Divide(x=w514, y=w522) -> (x/y=w523:dbl)
                    n436 = Add(x=w523, y=0.3) -> (x+y=w516:dbl)
                    n437 = call "Time Delay22"("error in (no error)"=w519, "Delay Time (s)"=w516) -> ("error out"=w518:errorcluster)  [unwired: 9 in]
                  }
                  frame #3 {
                    n438 = Negate(x=w526) -> (-x=w527:i32)
                    n439 = Number To Decimal String(number=w527) -> (decimal integer string=w528:string)  [unwired: 1 in]
                    n440 = call "mDrive Send Command.vi"("Extra"=w528, "Command"=T2."Move to Relative Position", "VISA resource name"=w524) -> ("VISA resource name out"=w525:refnum<visa-resource-name>)  [unwired: 4 in, 2 out]
                  }
                  frame #4 {
                    n441 = call "Time Delay23"("error in (no error)"=w535, "Delay Time (s)"=w534) -> ("error out"=w533:errorcluster)  [unwired: 9 in]
                  }
                  frame #5 {
                    n442 = property on="R Backlash corr" class="Bool (strict)"("Val(Sgnl)"=FALSE ("Value (Signaling)")) -> ()  [unwired: 2 in, 2 out]
                  }
                }
              }
              frame #1 {
              }
            }
          }
          frame #4 {
            n443 = property on="R Step PV" class="DigNum (strict)"() -> ("Value"=w550:i32)  [unwired: 2 in, 2 out]
            n444 = property on="R Step PV" class="DigNum (strict)"() -> ("Value"=w548:i32)  [unwired: 2 in, 2 out]
            n445 = property on="R steps/rev" class="DigNum (strict)"() -> ("Value"=w552:u32)  [unwired: 2 in, 2 out]
            n446 = To Double Precision Float(number=w552) -> (double precision float=w546:dbl)
            n447 = property on="R Step SP" class="DigNum (strict)"() -> ("Maximum"=w557:dbl)  [unwired: 2 in, 2 out]
            n448 = property on="R Step SP" class="DigNum (strict)"() -> ("Minimum"=w558:dbl)  [unwired: 2 in, 2 out]
            n449 = To Double Precision Float(number=w548) -> (double precision float=w547:dbl)
            n450 = To Double Precision Float(number=w550) -> (double precision float=w549:dbl)
            n451 = Subtract(x=w557, y=w549) -> (x-y=w556:dbl)
            n452 = Subtract(x=w558, y=w547) -> (x-y=w559:dbl)
            n453 = property on="R Velocity SP step/sec" class="DigNum (strict)"() -> ("Value"=w545:i32)  [unwired: 2 in, 2 out]
            n454 = property on="R Scan Length SP steps" class="DigNum (strict)"() -> ("Value"=w554:i32)  [unwired: 2 in, 2 out]
            n455 = To Double Precision Float(number=w554) -> (double precision float=w553:dbl)
            n456 = To Double Precision Float(number=w545) -> (double precision float=w544:dbl)
            n457 = property on="R Scan Length SP steps" class="DigNum (strict)"("Maximum"=w556) -> ()  [unwired: 2 in, 2 out]
            n458 = property on="R Scan Length SP steps" class="DigNum (strict)"("Minimum"=w559) -> ()  [unwired: 2 in, 2 out]
            n459 = Divide(x=w553, y=w546) -> (x/y=w555:dbl)
            n460 = Divide(x=w544, y=w546) -> (x/y=w543:dbl)
            n461 = property on="R deg/rev" class="DigNum (strict)"() -> ("Value"=w551:dbl)  [unwired: 2 in, 2 out]
            n462 = Multiply(x=w555, y=w551) -> (x*y=w542:dbl)
            n463 = Multiply(x=w551, y=w543) -> (x*y=w541:dbl)
            n464 = property on="R Scan length MV deg" class="DigNum (strict)"("Value"=w542) -> ()  [unwired: 2 in, 2 out]
            n465 = property on="R Scan Velocity SP deg/sec" class="DigNum (strict)"("Val(Sgnl)"=w541) -> ()  [unwired: 2 in, 2 out]
          }
        }
      }
      event #1 {
        n466 = event-data() -> ()  [unwired: 1 in, 5 out]
        n467 = property on="X Step SP" class="DigNum (strict)"() -> ("Value"=w1009:i32)  [unwired: 2 in, 2 out]
        n468 = property on="X steps/rev" class="DigNum (strict)"() -> ("Value"=w1007:u32)  [unwired: 2 in, 2 out]
        n469 = property on="X offset mm" class="DigNum (strict)"() -> ("Value"=w1005:dbl)  [unwired: 2 in, 2 out]
        n470 = To Double Precision Float(number=w1009) -> (double precision float=w1010:dbl)
        n471 = To Double Precision Float(number=w1007) -> (double precision float=w1013:dbl)
        n472 = Divide(x=w1010, y=w1013) -> (x/y=w1012:dbl)
        n473 = property on="X mm/rev" class="DigNum (strict)"() -> ("Value"=w1006:dbl)  [unwired: 2 in, 2 out]
        n474 = Multiply(x=w1012, y=w1006) -> (x*y=w1011:dbl)
        n475 = Add(x=w1011, y=w1005) -> (x+y=w1008:dbl)
        n476 = property on="X Position MV mm" class="DigNum (strict)"("Val(Sgnl)"=w1008) -> ()  [unwired: 2 in, 2 out]
      }
      event #2 {
        n477 = event-data() -> ()  [unwired: 1 in, 5 out]
        n478 = property on="Y steps/rev" class="DigNum (strict)"() -> ("Value"=w1016:u32)  [unwired: 2 in, 2 out]
        n479 = property on="Y offset mm" class="DigNum (strict)"() -> ("Value"=w1014:dbl)  [unwired: 2 in, 2 out]
        n480 = property on="Reset Y Position mm" class="DigNum (strict)"() -> ("Value"=w1022:dbl)  [unwired: 2 in, 2 out]
        n481 = Subtract(x=w1022, y=w1014) -> (x-y=w1021:dbl)
        n482 = property on="Y mm/rev" class="DigNum (strict)"() -> ("Value"=w1015:dbl)  [unwired: 2 in, 2 out]
        n483 = Divide(x=w1021, y=w1015) -> (x/y=w1020:dbl)
        n484 = To Double Precision Float(number=w1016) -> (double precision float=w1019:dbl)
        n485 = Multiply(x=w1020, y=w1019) -> (x*y=w1018:dbl)
        n486 = To Long Integer(number=w1018) -> (32bit integer=w1017:i32)
        n487 = property on="Reset Y Motor Steps" class="DigNum (strict)"("Val(Sgnl)"=w1017) -> ()  [unwired: 2 in, 2 out]
      }
      event #3 {
        n488 = event-data() -> ()  [unwired: 1 in, 5 out]
        n489 = property on="Y Step SP" class="DigNum (strict)"() -> ("Value"=w1027:i32)  [unwired: 2 in, 2 out]
        n490 = property on="Y steps/rev" class="DigNum (strict)"() -> ("Value"=w1025:u32)  [unwired: 2 in, 2 out]
        n491 = property on="Y offset mm" class="DigNum (strict)"() -> ("Value"=w1023:dbl)  [unwired: 2 in, 2 out]
        n492 = To Double Precision Float(number=w1027) -> (double precision float=w1028:dbl)
        n493 = To Double Precision Float(number=w1025) -> (double precision float=w1031:dbl)
        n494 = Divide(x=w1028, y=w1031) -> (x/y=w1030:dbl)
        n495 = property on="Y mm/rev" class="DigNum (strict)"() -> ("Value"=w1024:dbl)  [unwired: 2 in, 2 out]
        n496 = Multiply(x=w1030, y=w1024) -> (x*y=w1029:dbl)
        n497 = Add(x=w1029, y=w1023) -> (x+y=w1026:dbl)
        n498 = property on="Y Position MV mm" class="DigNum (strict)"("Val(Sgnl)"=w1026) -> ()  [unwired: 2 in, 2 out]
      }
      event #4 {
        n499 = event-data() -> ()  [unwired: 1 in, 5 out]
        n500 = property on="X Step SP" class="DigNum (strict)"() -> ("Value"=w1036:i32)  [unwired: 2 in, 2 out]
        n501 = property on="X steps/rev" class="DigNum (strict)"() -> ("Value"=w1034:u32)  [unwired: 2 in, 2 out]
        n502 = property on="X offset mm" class="DigNum (strict)"() -> ("Value"=w1032:dbl)  [unwired: 2 in, 2 out]
        n503 = To Double Precision Float(number=w1036) -> (double precision float=w1037:dbl)
        n504 = To Double Precision Float(number=w1034) -> (double precision float=w1040:dbl)
        n505 = Divide(x=w1037, y=w1040) -> (x/y=w1039:dbl)
        n506 = property on="X mm/rev" class="DigNum (strict)"() -> ("Value"=w1033:dbl)  [unwired: 2 in, 2 out]
        n507 = Multiply(x=w1039, y=w1033) -> (x*y=w1038:dbl)
        n508 = Add(x=w1038, y=w1032) -> (x+y=w1035:dbl)
        n509 = property on="X Position MV mm" class="DigNum (strict)"("Val(Sgnl)"=w1035) -> ()  [unwired: 2 in, 2 out]
      }
      event #5 {
        n510 = event-data() -> ()  [unwired: 1 in, 5 out]
        n511 = property on="Y steps/rev" class="DigNum (strict)"() -> ("Value"=w1042:u32)  [unwired: 2 in, 2 out]
        n512 = property on="Y Velocity SP step/sec" class="DigNum (strict)"() -> ("Value"=w1044:i32)  [unwired: 2 in, 2 out]
        n513 = To Double Precision Float(number=w1044) -> (double precision float=w1045:dbl)
        n514 = To Double Precision Float(number=w1042) -> (double precision float=w1047:dbl)
        n515 = Divide(x=w1045, y=w1047) -> (x/y=w1046:dbl)
        n516 = property on="Y mm/rev" class="DigNum (strict)"() -> ("Value"=w1041:dbl)  [unwired: 2 in, 2 out]
        n517 = Multiply(x=w1046, y=w1041) -> (x*y=w1043:dbl)
        n518 = property on="Y Velocity MV mm/sec" class="DigNum (strict)"("Val(Sgnl)"=w1043) -> ()  [unwired: 2 in, 2 out]
      }
      event #6 {
        n519 = event-data() -> ()  [unwired: 1 in, 5 out]
        n520 = property on="X steps/rev" class="DigNum (strict)"() -> ("Value"=w1049:u32)  [unwired: 2 in, 2 out]
        n521 = property on="X Velocity SP step/sec" class="DigNum (strict)"() -> ("Value"=w1051:i32)  [unwired: 2 in, 2 out]
        n522 = To Double Precision Float(number=w1051) -> (double precision float=w1052:dbl)
        n523 = To Double Precision Float(number=w1049) -> (double precision float=w1054:dbl)
        n524 = Divide(x=w1052, y=w1054) -> (x/y=w1053:dbl)
        n525 = property on="X mm/rev" class="DigNum (strict)"() -> ("Value"=w1048:dbl)  [unwired: 2 in, 2 out]
        n526 = Multiply(x=w1053, y=w1048) -> (x*y=w1050:dbl)
        n527 = property on="X Velocity MV mm/sec" class="DigNum (strict)"("Val(Sgnl)"=w1050) -> ()  [unwired: 2 in, 2 out]
      }
      event #7 {
        n528 = event-data() -> ()  [unwired: 1 in, 7 out]
        n529 = flat-sequence {
          frame #0 {
            n530 = property on="Y steps/rev" class="DigNum (strict)"() -> ("Value"=w1062:u32)  [unwired: 2 in, 2 out]
            n531 = property on="Y offset mm" class="DigNum (strict)"() -> ("Value"=w1060:dbl)  [unwired: 2 in, 2 out]
            n532 = property on="Y Position SP mm" class="DigNum (strict)"() -> ("Value"=w1059:dbl)  [unwired: 2 in, 2 out]
            n533 = Subtract(x=w1059, y=w1060) -> (x-y=w1064:dbl)
            n534 = property on="Y mm/rev" class="DigNum (strict)"() -> ("Value"=w1063:dbl)  [unwired: 2 in, 2 out]
            n535 = Divide(x=w1064, y=w1063) -> (x/y=w1065:dbl)
            n536 = To Double Precision Float(number=w1062) -> (double precision float=w1066:dbl)
            n537 = Multiply(x=w1065, y=w1066) -> (x*y=w1058:dbl)
            n538 = property on="Y Step SP" class="DigNum (strict)"() -> ("Maximum"=w1056:dbl)  [unwired: 2 in, 2 out]
            n539 = property on="Y Step SP" class="DigNum (strict)"() -> ("Minimum"=w1055:dbl)  [unwired: 2 in, 2 out]
            n540 = In Range and Coerce(upper limit=w1056, x=w1058, lower limit=w1055) -> (coerced(x)=w1057:dbl)  [unwired: 1 out]
            n541 = To Long Integer(number=w1057) -> (32bit integer=w1061:i32)
            n542 = property on="Y Step SP" class="DigNum (strict)"("Val(Sgnl)"=w1061) -> ()  [unwired: 2 in, 2 out]
          }
          frame #1 {
            n543 = property on="Y steps/rev" class="DigNum (strict)"() -> ("Value"=w1072:u32)  [unwired: 2 in, 2 out]
            n544 = To Double Precision Float(number=w1072) -> (double precision float=w1073:dbl)
            n545 = property on="Y Velocity SP step/sec" class="DigNum (strict)"() -> ("Maximum"=w1068:dbl)  [unwired: 2 in, 2 out]
            n546 = property on="Y Velocity SP step/sec" class="DigNum (strict)"() -> ("Minimum"=w1067:dbl)  [unwired: 2 in, 2 out]
            n547 = property on="Y Velocity SP mm/sec" class="DigNum (strict)"() -> ("Value"=w1074:dbl)  [unwired: 2 in, 2 out]
            n548 = property on="Y mm/rev" class="DigNum (strict)"() -> ("Value"=w1076:dbl)  [unwired: 2 in, 2 out]
            n549 = Divide(x=w1074, y=w1076) -> (x/y=w1075:dbl)
            n550 = Multiply(x=w1075, y=w1073) -> (x*y=w1070:dbl)
            n551 = In Range and Coerce(upper limit=w1068, x=w1070, lower limit=w1067) -> (coerced(x)=w1069:dbl)  [unwired: 1 out]
            n552 = To Long Integer(number=w1069) -> (32bit integer=w1071:i32)
            n553 = property on="Y Velocity SP step/sec" class="DigNum (strict)"("Val(Sgnl)"=w1071) -> ()  [unwired: 2 in, 2 out]
          }
        }
      }
      event #8 {
        n554 = event-data() -> ()  [unwired: 1 in, 7 out]
        n555 = flat-sequence {
          frame #0 {
            n556 = property on="X steps/rev" class="DigNum (strict)"() -> ("Value"=w1084:u32)  [unwired: 2 in, 2 out]
            n557 = To Double Precision Float(number=w1084) -> (double precision float=w1088:dbl)
            n558 = property on="X offset mm" class="DigNum (strict)"() -> ("Value"=w1082:dbl)  [unwired: 2 in, 2 out]
            n559 = property on="X Position SP mm" class="DigNum (strict)"() -> ("Value"=w1081:dbl)  [unwired: 2 in, 2 out]
            n560 = Subtract(x=w1081, y=w1082) -> (x-y=w1086:dbl)
            n561 = property on="X mm/rev" class="DigNum (strict)"() -> ("Value"=w1085:dbl)  [unwired: 2 in, 2 out]
            n562 = Divide(x=w1086, y=w1085) -> (x/y=w1087:dbl)
            n563 = Multiply(x=w1087, y=w1088) -> (x*y=w1080:dbl)
            n564 = property on="X Step SP" class="DigNum (strict)"() -> ("Maximum"=w1078:dbl)  [unwired: 2 in, 2 out]
            n565 = property on="X Step SP" class="DigNum (strict)"() -> ("Minimum"=w1077:dbl)  [unwired: 2 in, 2 out]
            n566 = In Range and Coerce(upper limit=w1078, x=w1080, lower limit=w1077) -> (coerced(x)=w1079:dbl)  [unwired: 1 out]
            n567 = To Long Integer(number=w1079) -> (32bit integer=w1083:i32)
            n568 = property on="X Step SP" class="DigNum (strict)"("Val(Sgnl)"=w1083) -> ()  [unwired: 2 in, 2 out]
          }
          frame #1 {
            n569 = property on="X steps/rev" class="DigNum (strict)"() -> ("Value"=w1094:u32)  [unwired: 2 in, 2 out]
            n570 = To Double Precision Float(number=w1094) -> (double precision float=w1095:dbl)
            n571 = property on="X Velocity SP step/sec" class="DigNum (strict)"() -> ("Maximum"=w1090:dbl)  [unwired: 2 in, 2 out]
            n572 = property on="X Velocity SP step/sec" class="DigNum (strict)"() -> ("Minimum"=w1089:dbl)  [unwired: 2 in, 2 out]
            n573 = property on="X Scan Velocity SP mm/sec" class="DigNum (strict)"() -> ("Value"=w1096:dbl)  [unwired: 2 in, 2 out]
            n574 = property on="X mm/rev" class="DigNum (strict)"() -> ("Value"=w1098:dbl)  [unwired: 2 in, 2 out]
            n575 = Divide(x=w1096, y=w1098) -> (x/y=w1097:dbl)
            n576 = Multiply(x=w1097, y=w1095) -> (x*y=w1092:dbl)
            n577 = In Range and Coerce(upper limit=w1090, x=w1092, lower limit=w1089) -> (coerced(x)=w1091:dbl)  [unwired: 1 out]
            n578 = To Long Integer(number=w1091) -> (32bit integer=w1093:i32)
            n579 = property on="X Velocity SP step/sec" class="DigNum (strict)"("Val(Sgnl)"=w1093) -> ()  [unwired: 2 in, 2 out]
          }
        }
      }
      event #9 {
        n580 = event-data() -> ()  [unwired: 1 in, 7 out]
        n581 = flat-sequence {
          frame #0 {
            n582 = property on="Y steps/rev" class="DigNum (strict)"() -> ("Value"=w1105:u32)  [unwired: 2 in, 2 out]
            n583 = To Double Precision Float(number=w1105) -> (double precision float=w1108:dbl)
            n584 = property on="Y Scan Length SP mm" class="DigNum (strict)"() -> ("Value"=w1103:dbl)  [unwired: 2 in, 2 out]
            n585 = property on="Y mm/rev" class="DigNum (strict)"() -> ("Value"=w1106:dbl)  [unwired: 2 in, 2 out]
            n586 = Divide(x=w1103, y=w1106) -> (x/y=w1107:dbl)
            n587 = Multiply(x=w1107, y=w1108) -> (x*y=w1102:dbl)
            n588 = property on="Y Step SP" class="DigNum (strict)"() -> ("Maximum"=w1099:dbl)  [unwired: 2 in, 2 out]
            n589 = property on="Y Step SP" class="DigNum (strict)"() -> ("Minimum"=w1100:dbl)  [unwired: 2 in, 2 out]
            n590 = In Range and Coerce(upper limit=w1099, x=w1102, lower limit=w1100) -> (coerced(x)=w1101:dbl)  [unwired: 1 out]
            n591 = To Long Integer(number=w1101) -> (32bit integer=w1104:i32)
            n592 = property on="Y Scan Length SP steps" class="DigNum (strict)"("Val(Sgnl)"=w1104) -> ()  [unwired: 2 in, 2 out]
          }
          frame #1 {
            n593 = property on="Y steps/rev" class="DigNum (strict)"() -> ("Value"=w1114:u32)  [unwired: 2 in, 2 out]
            n594 = To Double Precision Float(number=w1114) -> (double precision float=w1115:dbl)
            n595 = property on="Y Scan Velocity SP mm/sec" class="DigNum (strict)"() -> ("Value"=w1116:dbl)  [unwired: 2 in, 2 out]
            n596 = property on="Y Scan Velocity SP steps/sec" class="DigNum (strict)"() -> ("Maximum"=w1110:dbl)  [unwired: 2 in, 2 out]
            n597 = property on="Y Scan Velocity SP steps/sec" class="DigNum (strict)"() -> ("Minimum"=w1109:dbl)  [unwired: 2 in, 2 out]
            n598 = property on="Y mm/rev" class="DigNum (strict)"() -> ("Value"=w1118:dbl)  [unwired: 2 in, 2 out]
            n599 = Divide(x=w1116, y=w1118) -> (x/y=w1117:dbl)
            n600 = Multiply(x=w1117, y=w1115) -> (x*y=w1112:dbl)
            n601 = In Range and Coerce(upper limit=w1110, x=w1112, lower limit=w1109) -> (coerced(x)=w1111:dbl)  [unwired: 1 out]
            n602 = To Long Integer(number=w1111) -> (32bit integer=w1113:i32)
            n603 = property on="Y Scan Velocity SP steps/sec" class="DigNum (strict)"("Val(Sgnl)"=w1113) -> ()  [unwired: 2 in, 2 out]
          }
        }
      }
      event #10 {
        n604 = event-data() -> ()  [unwired: 1 in, 7 out]
        n605 = flat-sequence {
          frame #0 {
            n606 = property on="X steps/rev" class="DigNum (strict)"() -> ("Value"=w1125:u32)  [unwired: 2 in, 2 out]
            n607 = To Double Precision Float(number=w1125) -> (double precision float=w1128:dbl)
            n608 = property on="X Scan Length SP mm" class="DigNum (strict)"() -> ("Value"=w1123:dbl)  [unwired: 2 in, 2 out]
            n609 = property on="X mm/rev" class="DigNum (strict)"() -> ("Value"=w1126:dbl)  [unwired: 2 in, 2 out]
            n610 = Divide(x=w1123, y=w1126) -> (x/y=w1127:dbl)
            n611 = Multiply(x=w1127, y=w1128) -> (x*y=w1122:dbl)
            n612 = property on="X Step SP" class="DigNum (strict)"() -> ("Maximum"=w1119:dbl)  [unwired: 2 in, 2 out]
            n613 = property on="X Step SP" class="DigNum (strict)"() -> ("Minimum"=w1120:dbl)  [unwired: 2 in, 2 out]
            n614 = In Range and Coerce(upper limit=w1119, x=w1122, lower limit=w1120) -> (coerced(x)=w1121:dbl)  [unwired: 1 out]
            n615 = To Long Integer(number=w1121) -> (32bit integer=w1124:i32)
            n616 = property on="X Scan Length SP steps" class="DigNum (strict)"("Val(Sgnl)"=w1124) -> ()  [unwired: 2 in, 2 out]
          }
          frame #1 {
            n617 = property on="X steps/rev" class="DigNum (strict)"() -> ("Value"=w1134:u32)  [unwired: 2 in, 2 out]
            n618 = To Double Precision Float(number=w1134) -> (double precision float=w1135:dbl)
            n619 = property on="X Scan Velocity SP mm/sec" class="DigNum (strict)"() -> ("Value"=w1136:dbl)  [unwired: 2 in, 2 out]
            n620 = property on="X Scan Velocity SP steps/sec" class="DigNum (strict)"() -> ("Maximum"=w1130:dbl)  [unwired: 2 in, 2 out]
            n621 = property on="X Scan Velocity SP steps/sec" class="DigNum (strict)"() -> ("Minimum"=w1129:dbl)  [unwired: 2 in, 2 out]
            n622 = property on="X mm/rev" class="DigNum (strict)"() -> ("Value"=w1138:dbl)  [unwired: 2 in, 2 out]
            n623 = Divide(x=w1136, y=w1138) -> (x/y=w1137:dbl)
            n624 = Multiply(x=w1137, y=w1135) -> (x*y=w1132:dbl)
            n625 = In Range and Coerce(upper limit=w1130, x=w1132, lower limit=w1129) -> (coerced(x)=w1131:dbl)  [unwired: 1 out]
            n626 = To Long Integer(number=w1131) -> (32bit integer=w1133:i32)
            n627 = property on="X Scan Velocity SP steps/sec" class="DigNum (strict)"("Val(Sgnl)"=w1133) -> ()  [unwired: 2 in, 2 out]
          }
        }
      }
      event #11 {
        n628 = event-data() -> ()  [unwired: 1 in, 7 out]
        n629 = flat-sequence {
          tunnel: w1143 -> [w1153]
          tunnel: w1144 -> [w1154]
          tunnel: [w1154] -> w1140
          tunnel: [w1153] -> w1139
          tunnel: [w1157] -> w1142
          tunnel: [w1156] -> w1141
          tunnel: w1140 -> [w1159]
          tunnel: w1139 -> [w1158]
          tunnel: [w1177] -> w1146
          tunnel: [w1176] -> w1145
          tunnel: w1142 -> [w1175]
          tunnel: w1141 -> [w1174]
          tunnel: [w1184] -> w1148
          tunnel: [w1183] -> w1147
          tunnel: w1146 -> [w1182]
          tunnel: w1145 -> [w1181]
          tunnel: [w1190] -> w1149
          tunnel: [w1191] -> w1150
          tunnel: w1148 -> [w1191]
          tunnel: w1147 -> [w1189]
          frame #0 {
            n630 = property on="Y Go" class="Bool"("DisabledEnum"=T1."Disabled and Grayed Out" ("Disabled")) -> ()  [unwired: 2 in, 2 out]
            n631 = property on="Scan Go" class="Bool"("DisabledEnum"=T1."Disabled and Grayed Out" ("Disabled")) -> ()  [unwired: 2 in, 2 out]
          }
          frame #1 {
            n632 = property on="Y Step SP" class="DigNum (strict)"() -> ("Value"=w1167:i32)  [unwired: 2 in, 2 out]
            n633 = property on="Y Step PV" class="DigNum (strict)"() -> ("Value"=w1166:i32)  [unwired: 2 in, 2 out]
            n634 = property on="Y Backlash" class="DigNum (strict)"() -> ("Value"=w1155:i32)  [unwired: 2 in, 2 out]
            n635 = Subtract(x=w1167, y=w1166) -> (x-y=w1165:i32)
            n636 = Sign(1:w1155) -> (0:w1163:i32)
            n637 = Sign(1:w1165) -> (0:w1164:i32)
            n638 = Multiply(x=w1164, y=w1163) -> (x*y=w1162:i32)
            n639 = Equal?(x=w1162, y=1) -> (x = y?=w1160:bool)
            n640 = case shown="False" w1160 {
              tunnel: w1159 -> [w1170 w1172]
              tunnel: w1158 -> [w1169 w1171]
              tunnel: [w1169 w1171] -> w1157
              tunnel: [w1170 w1172] -> w1156
              frame #0 {
                n641 = property on="Y Backlash corr" class="Bool (strict)"("Val(Sgnl)"=FALSE ("Value (Signaling)")) -> ()  [unwired: 2 in, 2 out]
              }
              frame #1 {
                n642 = property on="Y Backlash corr" class="Bool (strict)"("Val(Sgnl)"=TRUE ("Value (Signaling)")) -> ()  [unwired: 2 in, 2 out]
              }
            }
          }
          frame #2 {
            # "Velocity Setting"
            n643 = property on="Y Velocity SP step/sec" class="DigNum (strict)"() -> ("Value"=w1178:i32)  [unwired: 2 in, 2 out]
            n644 = Number To Decimal String(number=w1178) -> (decimal integer string=w1179:string)  [unwired: 1 in]
            n645 = call "mDrive Send Command.vi"("error in (no error)"=w1175, "Extra"=w1179, "Command"=T2."Max Velocity", "VISA resource name"=w1174) -> ("error out"=w1176:errorcluster, "VISA resource name out"=w1177:refnum<visa-resource-name>)  [unwired: 3 in, 1 out]
          }
          frame #3 {
            # "Move to Abs Position"
            n646 = property on="Y Step SP" class="DigNum (strict)"() -> ("Value"=w1187:i32)  [unwired: 2 in, 2 out]
            n647 = Number To Decimal String(number=w1187) -> (decimal integer string=w1186:string)  [unwired: 1 in]
            n648 = call "mDrive Send Command.vi"("error in (no error)"=w1181, "Extra"=w1186, "Command"=T2."Move to Absolute Position", "VISA resource name"=w1182) -> ("error out"=w1183:errorcluster, "VISA resource name out"=w1184:refnum<visa-resource-name>)  [unwired: 3 in, 1 out]
          }
          frame #4 {
            n649 = call "Time Delay"("error in (no error)"=w1189, "Delay Time (s)"=0.1) -> ("error out"=w1190:errorcluster)  [unwired: 9 in]
          }
        }
      }
      event #12 {
        n650 = event-data() -> ()  [unwired: 1 in, 7 out]
        n651 = flat-sequence {
          tunnel: [w1205] -> w1197
          tunnel: [w1204] -> w1196
          tunnel: w1195 -> [w1205]
          tunnel: w1194 -> [w1204]
          tunnel: [w1210] -> w1199
          tunnel: [w1209] -> w1198
          tunnel: w1197 -> [w1212]
          tunnel: w1196 -> [w1211]
          tunnel: [w1230] -> w1201
          tunnel: [w1229] -> w1200
          tunnel: w1199 -> [w1228]
          tunnel: w1198 -> [w1227]
          tunnel: [w1237] -> w1203
          tunnel: [w1236] -> w1202
          tunnel: w1201 -> [w1235]
          tunnel: w1200 -> [w1234]
          tunnel: [w1243] -> w1192
          tunnel: [w1244] -> w1193
          tunnel: w1203 -> [w1244]
          tunnel: w1202 -> [w1242]
          frame #0 {
            n652 = property on="X Go" class="Bool"("DisabledEnum"=T1."Disabled and Grayed Out" ("Disabled")) -> ()  [unwired: 2 in, 2 out]
            n653 = property on="Scan Go" class="Bool"("DisabledEnum"=T1."Disabled and Grayed Out" ("Disabled")) -> ()  [unwired: 2 in, 2 out]
          }
          frame #1 {
            n654 = property on="X Step SP" class="DigNum (strict)"() -> ("Value"=w1220:i32)  [unwired: 2 in, 2 out]
            n655 = property on="X Step PV" class="DigNum (strict)"() -> ("Value"=w1219:i32)  [unwired: 2 in, 2 out]
            n656 = property on="X Backlash" class="DigNum (strict)"() -> ("Value"=w1208:i32)  [unwired: 2 in, 2 out]
            n657 = Subtract(x=w1220, y=w1219) -> (x-y=w1218:i32)
            n658 = Sign(1:w1208) -> (0:w1216:i32)
            n659 = Sign(1:w1218) -> (0:w1217:i32)
            n660 = Multiply(x=w1217, y=w1216) -> (x*y=w1215:i32)
            n661 = Equal?(x=w1215, y=1) -> (x = y?=w1213:bool)
            n662 = case shown="False" w1213 {
              tunnel: w1212 -> [w1223 w1225]
              tunnel: w1211 -> [w1222 w1224]
              tunnel: [w1222 w1224] -> w1210
              tunnel: [w1223 w1225] -> w1209
              frame #0 {
                n663 = property on="X Backlash corr" class="Bool (strict)"("Val(Sgnl)"=FALSE ("Value (Signaling)")) -> ()  [unwired: 2 in, 2 out]
              }
              frame #1 {
                n664 = property on="Y Backlash corr" class="Bool (strict)"("Val(Sgnl)"=TRUE ("Value (Signaling)")) -> ()  [unwired: 2 in, 2 out]
              }
            }
          }
          frame #2 {
            # "Velocity Setting"
            n665 = property on="X Scan Velocity SP steps/sec" class="DigNum (strict)"() -> ("Value"=w1231:i32)  [unwired: 2 in, 2 out]
            n666 = Number To Decimal String(number=w1231) -> (decimal integer string=w1232:string)  [unwired: 1 in]
            n667 = call "mDrive Send Command.vi"("error in (no error)"=w1228, "Extra"=w1232, "Command"=T2."Max Velocity", "VISA resource name"=w1227) -> ("error out"=w1229:errorcluster, "VISA resource name out"=w1230:refnum<visa-resource-name>)  [unwired: 3 in, 1 out]
          }
          frame #3 {
            # "Move to Abs Position"
            n668 = property on="X Step SP" class="DigNum (strict)"() -> ("Value"=w1240:i32)  [unwired: 2 in, 2 out]
            n669 = Number To Decimal String(number=w1240) -> (decimal integer string=w1239:string)  [unwired: 1 in]
            n670 = call "mDrive Send Command.vi"("error in (no error)"=w1234, "Extra"=w1239, "Command"=T2."Move to Absolute Position", "VISA resource name"=w1235) -> ("error out"=w1236:errorcluster, "VISA resource name out"=w1237:refnum<visa-resource-name>)  [unwired: 3 in, 1 out]
          }
          frame #4 {
            n671 = call "Time Delay15"("error in (no error)"=w1242, "Delay Time (s)"=0.1) -> ("error out"=w1243:errorcluster)  [unwired: 9 in]
          }
        }
      }
      event #13 {
        n672 = event-data() -> ()  [unwired: 1 in, 7 out]
        n673 = flat-sequence {
          tunnel: [w1260] -> w1252
          tunnel: [w1258] -> w1251
          tunnel: w1250 -> [w1254]
          tunnel: w1249 -> [w1253]
          tunnel: w1252 -> [w1275]
          tunnel: w1251 -> [w1274]
          tunnel: [w1275] -> w1246
          tunnel: [w1274] -> w1245
          tunnel: [w1278] -> w1247
          tunnel: [w1279] -> w1248
          tunnel: w1246 -> [w1279]
          tunnel: w1245 -> [w1278]
          frame #0 {
            # "VELOCITY"
            n674 = property on="X Scan Velocity SP steps/sec" class="DigNum (strict)"() -> ("Value"=w1261:i32)  [unwired: 2 in, 2 out]
            n675 = Number To Decimal String(number=w1261) -> (decimal integer string=w1262:string)  [unwired: 1 in]
            n676 = call "mDrive Send Command.vi"("error in (no error)"=w1253, "Extra"=w1262, "Command"=T2."Max Velocity", "VISA resource name"=w1254) -> ("error out"=w1263:errorcluster, "VISA resource name out"=w1268:refnum<visa-resource-name>)  [unwired: 3 in, 1 out]
            n677 = call "Time Delay9"("error in (no error)"=w1263) -> ("error out"=w1266:errorcluster)  [unwired: 10 in]
            n678 = call "mDrive Send Command.vi"("error in (no error)"=w1266, "Extra"="VM", "Command"=T2."Print Parameter", "VISA resource name"=w1268) -> ("error out"=w1259:errorcluster, "read buffer"=w1264:string, "VISA resource name out"=w1260:refnum<visa-resource-name>)  [unwired: 3 in]
            n679 = call "Time Delay10"("error in (no error)"=w1259) -> ("error out"=w1258:errorcluster)  [unwired: 10 in]
            n680 = Decimal String To Number(string=w1264, offset=0) -> (number=w1267:i32)  [unwired: 1 in, 1 out]
            n681 = property on="X velocity PV step/sec" class="DigNum (strict)"("Val(Sgnl)"=w1267) -> ()  [unwired: 2 in, 2 out]
          }
          frame #1 {
            n682 = property on="X Scan" class="Bool (strict)"("Val(Sgnl)"=TRUE ("Slew Ready 2")) -> ()  [unwired: 2 in, 2 out]
            n683 = property on="Scan Go" class="Bool"("DisabledEnum"=T1."Enabled" ("Disabled")) -> ()  [unwired: 2 in, 2 out]
            n684 = property on="Scan Cancel" class="Bool"("DisabledEnum"=T1."Enabled" ("Disabled")) -> ()  [unwired: 2 in, 2 out]
            n685 = property on="X Scan Length SP steps" class="DigNum (strict)"("DisabledEnum"=T1."Disabled and Grayed Out" ("Disabled")) -> ()  [unwired: 2 in, 2 out]
            n686 = property on="X Scan Velocity SP steps/sec" class="DigNum (strict)"("DisabledEnum"=T1."Disabled and Grayed Out" ("Disabled")) -> ()  [unwired: 2 in, 2 out]
          }
          frame #2 {
            n687 = property on="X Go" class="Bool"("DisabledEnum"=T1."Disabled and Grayed Out" ("Disabled")) -> ()  [unwired: 2 in, 2 out]
            n688 = property on="Y Go" class="Bool"("DisabledEnum"=T1."Disabled and Grayed Out" ("Disabled")) -> ()  [unwired: 2 in, 2 out]
          }
        }
      }
      event #14 {
        n689 = event-data() -> ()  [unwired: 1 in, 7 out]
        n690 = flat-sequence {
          tunnel: w1287 -> [w1297]
          tunnel: w1286 -> [w1296]
          tunnel: [w1293] -> w1284
          tunnel: [w1291] -> w1283
          tunnel: w1284 -> [w1310]
          tunnel: w1283 -> [w1309]
          tunnel: [w1310] -> w1281
          tunnel: [w1309] -> w1280
          tunnel: [w1313] -> w1285
          tunnel: [w1314] -> w1282
          tunnel: w1281 -> [w1314]
          tunnel: w1280 -> [w1313]
          frame #0 {
            # "VELOCITY"
            n691 = property on="Y Scan Velocity SP steps/sec" class="DigNum (strict)"() -> ("Value"=w1294:i32)  [unwired: 2 in, 2 out]
            n692 = Number To Decimal String(number=w1294) -> (decimal integer string=w1295:string)  [unwired: 1 in]
            n693 = call "mDrive Send Command.vi"("error in (no error)"=w1297, "Extra"=w1295, "Command"=T2."Max Velocity", "VISA resource name"=w1296) -> ("error out"=w1298:errorcluster, "VISA resource name out"=w1303:refnum<visa-resource-name>)  [unwired: 3 in, 1 out]
            n694 = call "Time Delay5"("error in (no error)"=w1298) -> ("error out"=w1301:errorcluster)  [unwired: 10 in]
            n695 = call "mDrive Send Command.vi"("error in (no error)"=w1301, "Extra"="VM", "Command"=T2."Print Parameter", "VISA resource name"=w1303) -> ("error out"=w1292:errorcluster, "read buffer"=w1299:string, "VISA resource name out"=w1293:refnum<visa-resource-name>)  [unwired: 3 in]
            n696 = call "Time Delay6"("error in (no error)"=w1292) -> ("error out"=w1291:errorcluster)  [unwired: 10 in]
            n697 = Decimal String To Number(string=w1299, offset=0) -> (number=w1302:i32)  [unwired: 1 in, 1 out]
            n698 = property on="Y velocity PV step/sec" class="DigNum (strict)"("Val(Sgnl)"=w1302) -> ()  [unwired: 2 in, 2 out]
          }
          frame #1 {
            n699 = property on="Y Scan" class="Bool (strict)"("Val(Sgnl)"=TRUE ("Slew Ready 2")) -> ()  [unwired: 2 in, 2 out]
            n700 = property on="Scan Go" class="Bool"("DisabledEnum"=T1."Enabled" ("Disabled")) -> ()  [unwired: 2 in, 2 out]
            n701 = property on="Scan Cancel" class="Bool"("DisabledEnum"=T1."Enabled" ("Disabled")) -> ()  [unwired: 2 in, 2 out]
            n702 = property on="Y Scan Length SP steps" class="DigNum (strict)"("DisabledEnum"=T1."Disabled and Grayed Out" ("Disabled")) -> ()  [unwired: 2 in, 2 out]
            n703 = property on="Y Scan Velocity SP steps/sec" class="DigNum (strict)"("DisabledEnum"=T1."Disabled and Grayed Out" ("Disabled")) -> ()  [unwired: 2 in, 2 out]
          }
          frame #2 {
            n704 = property on="X Go" class="Bool"("DisabledEnum"=T1."Disabled and Grayed Out" ("Disabled")) -> ()  [unwired: 2 in, 2 out]
            n705 = property on="Y Go" class="Bool"("DisabledEnum"=T1."Disabled and Grayed Out" ("Disabled")) -> ()  [unwired: 2 in, 2 out]
          }
        }
      }
      event #15 {
        n706 = event-data() -> ()  [unwired: 1 in, 4 out]
        n707 = event-data() -> ()  [unwired: 3 in, 1 out]
      }
      event #16 {
        n708 = event-data() -> ()  [unwired: 1 in, 7 out]
        n709 = flat-sequence {
          tunnel: [w1342] -> w1323
          tunnel: [w1341] -> w1322
          tunnel: w1325 -> [w1340]
          tunnel: w1324 -> [w1339]
          frame #0 {
            n710 = call "mDrive Send Command.vi"("error in (no error)"=w1339, "Command"=T2."Stop", "VISA resource name"=w1340) -> ("error out"=w1341:errorcluster, "VISA resource name out"=w1342:refnum<visa-resource-name>)  [unwired: 4 in, 1 out]
          }
        }
        n711 = flat-sequence {
          tunnel: [w1347] -> w1329
          tunnel: [w1346] -> w1328
          tunnel: w1327 -> [w1345]
          tunnel: w1326 -> [w1344]
          frame #0 {
            n712 = call "mDrive Send Command.vi"("error in (no error)"=w1344, "Command"=T2."Stop", "VISA resource name"=w1345) -> ("error out"=w1346:errorcluster, "VISA resource name out"=w1347:refnum<visa-resource-name>)  [unwired: 4 in, 1 out]
          }
        }
        n713 = flat-sequence {
          tunnel: w1333 -> [w1353]
          tunnel: w1332 -> [w1352]
          tunnel: [w1351] -> w1331
          tunnel: [w1350] -> w1330
          frame #0 {
            n714 = call "mDrive Send Command.vi"("error in (no error)"=w1352, "Command"=T2."Stop", "VISA resource name"=w1353) -> ("error out"=w1350:errorcluster, "VISA resource name out"=w1351:refnum<visa-resource-name>)  [unwired: 4 in, 1 out]
          }
        }
        n715 = flat-sequence {
          tunnel: w1321 -> [w1338]
          tunnel: w1320 -> [w1337]
          tunnel: [w1336] -> w1319
          tunnel: [w1334] -> _
          tunnel: [w1334] -> w1318
          frame #0 {
            n716 = call "mDrive Send Command.vi"("error in (no error)"=w1337, "Command"=T2."Stop", "VISA resource name"=w1338) -> ("error out"=w1334:errorcluster, "VISA resource name out"=w1336:refnum<visa-resource-name>)  [unwired: 4 in, 1 out]
          }
        }
      }
      event #17 {
        n717 = event-data() -> ()  [unwired: 1 in, 7 out]
        n718 = flat-sequence {
          tunnel: [w1378] -> w1359
          tunnel: [w1377] -> w1358
          tunnel: w1357 -> [w1375]
          tunnel: w1356 -> [w1374]
          tunnel: [w1385] -> w1354
          tunnel: [w1386] -> w1355
          tunnel: w1359 -> [w1386]
          tunnel: w1358 -> [w1385]
          frame #0 {
            n719 = call "mDrive Send Command.vi"("error in (no error)"=w1374, "Command"=T2."Stop", "VISA resource name"=w1375) -> ("error out"=w1377:errorcluster, "VISA resource name out"=w1378:refnum<visa-resource-name>)  [unwired: 4 in, 1 out]
          }
          frame #1 {
            n720 = property on="Z Scan" class="Bool (strict)"("Value"=FALSE ("Slew Ready")) -> ()  [unwired: 2 in, 2 out]
            n721 = property on="Z Scan set" class="Bool"("DisabledEnum"=T1."Enabled" ("Disabled")) -> ()  [unwired: 2 in, 2 out]
            n722 = property on="Z Scan Velocity SP steps/sec" class="DigNum (strict)"("DisabledEnum"=T1."Enabled" ("Disabled")) -> ()  [unwired: 2 in, 2 out]
            n723 = property on="Z Scan Length SP steps" class="DigNum (strict)"("DisabledEnum"=T1."Enabled" ("Disabled")) -> ()  [unwired: 2 in, 2 out]
            n724 = property on="Z Go" class="Bool"("DisabledEnum"=T1."Enabled" ("Disabled")) -> ()  [unwired: 2 in, 2 out]
            n725 = property on="Z Scan OK" class="Bool"("DisabledEnum"=T1."Enabled" ("Disabled")) -> ()  [unwired: 2 in, 2 out]
          }
        }
        n726 = flat-sequence {
          tunnel: w1363 -> [w1389]
          tunnel: w1362 -> [w1388]
          tunnel: [w1391] -> w1365
          tunnel: [w1390] -> w1364
          tunnel: [w1398] -> w1360
          tunnel: [w1399] -> w1361
          tunnel: w1365 -> [w1399]
          tunnel: w1364 -> [w1398]
          frame #0 {
            n727 = call "mDrive Send Command.vi"("error in (no error)"=w1388, "Command"=T2."Stop", "VISA resource name"=w1389) -> ("error out"=w1390:errorcluster, "VISA resource name out"=w1391:refnum<visa-resource-name>)  [unwired: 4 in, 1 out]
          }
          frame #1 {
            n728 = property on="X Scan" class="Bool (strict)"("Value"=FALSE ("Slew Ready")) -> ()  [unwired: 2 in, 2 out]
            n729 = property on="X Scan set" class="Bool"("DisabledEnum"=T1."Enabled" ("Disabled")) -> ()  [unwired: 2 in, 2 out]
            n730 = property on="X Scan Velocity SP steps/sec" class="DigNum (strict)"("DisabledEnum"=T1."Enabled" ("Disabled")) -> ()  [unwired: 2 in, 2 out]
            n731 = property on="X Scan Length SP steps" class="DigNum (strict)"("DisabledEnum"=T1."Enabled" ("Disabled")) -> ()  [unwired: 2 in, 2 out]
            n732 = property on="X Go" class="Bool"("DisabledEnum"=T1."Enabled" ("Disabled")) -> ()  [unwired: 2 in, 2 out]
            n733 = property on="X Scan OK" class="Bool"("DisabledEnum"=T1."Enabled" ("Disabled")) -> ()  [unwired: 2 in, 2 out]
          }
        }
        n734 = flat-sequence {
          tunnel: w1371 -> [w1402]
          tunnel: w1370 -> [w1401]
          tunnel: [w1404] -> w1367
          tunnel: [w1403] -> w1366
          tunnel: [w1411] -> w1372
          tunnel: [w1412] -> w1373
          tunnel: w1367 -> [w1412]
          tunnel: w1366 -> [w1411]
          frame #0 {
            n735 = call "mDrive Send Command.vi"("error in (no error)"=w1401, "Command"=T2."Stop", "VISA resource name"=w1402) -> ("error out"=w1403:errorcluster, "VISA resource name out"=w1404:refnum<visa-resource-name>)  [unwired: 4 in, 1 out]
          }
          frame #1 {
            n736 = property on="Y Scan" class="Bool (strict)"("Value"=FALSE ("Slew Ready")) -> ()  [unwired: 2 in, 2 out]
            n737 = property on="Y Scan Velocity SP steps/sec" class="DigNum (strict)"("DisabledEnum"=T1."Enabled" ("Disabled")) -> ()  [unwired: 2 in, 2 out]
            n738 = property on="Y Go" class="Bool"("DisabledEnum"=T1."Enabled" ("Disabled")) -> ()  [unwired: 2 in, 2 out]
            n739 = property on="Y Scan OK" class="Bool"("DisabledEnum"=T1."Enabled" ("Disabled")) -> ()  [unwired: 2 in, 2 out]
            n740 = property on="Y Scan Length SP steps" class="DigNum (strict)"("DisabledEnum"=T1."Enabled" ("Disabled")) -> ()  [unwired: 2 in, 2 out]
            n741 = property on="Y Scan OK" class="Bool"("DisabledEnum"=T1."Enabled" ("Disabled")) -> ()  [unwired: 2 in, 2 out]
          }
        }
        n742 = property on="Scan Go" class="Bool"("DisabledEnum"=T1."Disabled and Grayed Out" ("Disabled")) -> ()  [unwired: 2 in, 2 out]
        n743 = property on="Scan Cancel" class="Bool"("DisabledEnum"=T1."Disabled and Grayed Out" ("Disabled")) -> ()  [unwired: 2 in, 2 out]
      }
      event #18 {
        n744 = event-data() -> ()  [unwired: 1 in, 7 out]
        n745 = property on="Y Scan" class="Bool (strict)"() -> ("Value"=w1416:bool)  [unwired: 2 in, 2 out]
        n746 = flat-sequence {
          tunnel: w1429 -> [w1432]
          tunnel: w1428 -> [w1433]
          tunnel: [w1433] -> w1425
          tunnel: [w1432] -> w1424
          tunnel: [w1431] -> w1423
          tunnel: w1416 -> [w1430]
          tunnel: [w1430] -> w1415
          tunnel: w1425 -> [w1444]
          tunnel: [w1446] -> w1420
          tunnel: w1424 -> [w1443]
          tunnel: [w1445] -> w1418
          tunnel: w1423 -> [w1442]
          tunnel: w1415 -> [w1441]
          tunnel: [w1441] -> w1413
          tunnel: w1420 -> [w1457]
          tunnel: [w1457] -> w1419
          tunnel: w1418 -> [w1456]
          tunnel: [w1456] -> w1417
          tunnel: [w1454] -> w1414
          tunnel: w1413 -> [w1454]
          tunnel: w1419 -> [w1462]
          tunnel: [w1460] -> w1422
          tunnel: w1417 -> [w1461]
          tunnel: [w1459] -> w1421
          tunnel: w1414 -> [w1458]
          tunnel: w1422 -> [w1478]
          tunnel: w1421 -> [w1477]
          tunnel: [w1478] -> w1427
          tunnel: [w1477] -> w1426
          frame #0 {
            n747 = case shown="True" w1430 {
              tunnel: ["" w1435] -> w1431
              frame #0 {
              }
              frame #1 {
                n748 = property on="Y Scan Length SP steps" class="DigNum (strict)"() -> ("Value"=w1440:i32)  [unwired: 2 in, 2 out]
                n749 = Number To Decimal String(number=w1440) -> (decimal integer string=w1437:string)  [unwired: 1 in]
                n750 = call <vilib>:"Space Constant.vi"() -> ("String"=w1438:string)
                n751 = Concatenate Strings("MR", w1438, w1437, "\r") -> (w1435:string)
              }
            }
          }
          frame #1 {
            n752 = case shown="True" w1441 {
              tunnel: [w1448 w1453] -> w1446
              tunnel: [w1447 w1452] -> w1445
              tunnel: w1444 -> [w1448 w1451]
              tunnel: w1443 -> [w1447 w1450]
              tunnel: w1442 -> [_ w1449]
              frame #0 {
              }
              frame #1 {
                n753 = VISA Write(VISA resource name=w1451, write buffer=w1449, error in (no error)=w1450) -> (VISA resource name out=w1453:refnum<visa-resource-name>, error out=w1452:errorcluster)  [unwired: 1 out]
              }
            }
          }
          frame #2 {
            n754 = call "Time Delay7"("Delay Time (s)"=0.1) -> ()  [unwired: 10 in, 1 out]
          }
          frame #3 {
            n755 = case shown="True" w1458 {
              tunnel: w1462 -> [w1464 w1468]
              tunnel: w1461 -> [w1463 w1467]
              tunnel: [w1464 w1466] -> w1460
              tunnel: [w1463 w1465] -> w1459
              frame #0 {
              }
              frame #1 {
                n756 = property class="Instr"(reference=w1468, error in=w1467) -> (reference out=w1470:refnum<visa-resource-name>, error out=w1469:errorcluster, "Serial Settings:Number of Bytes at Serial Port"=w1471:u32)
                n757 = VISA Read(VISA resource name=w1470, byte count=w1471, error in (no error)=w1469) -> (VISA resource name out=w1466:refnum<visa-resource-name>, error out=w1465:errorcluster)  [unwired: 2 out]
              }
            }
          }
          frame #4 {
            n758 = property on="Y Scan" class="Bool (strict)"("Val(Sgnl)"=FALSE ("Slew Ready 2")) -> ()  [unwired: 2 in, 2 out]
            n759 = property on="Y Scan Length SP steps" class="DigNum (strict)"("DisabledEnum"=T1."Enabled" ("Disabled")) -> ()  [unwired: 2 in, 2 out]
            n760 = property on="Slew Velocity" class="DigNum (strict)"("DisabledEnum"=T1."Enabled" ("Disabled")) -> ()  [unwired: 2 in, 2 out]
            n761 = property on="Scan Cancel" class="Bool"("DisabledEnum"=T1."Disabled and Grayed Out" ("Disabled")) -> ()  [unwired: 2 in, 2 out]
            n762 = property on="Scan Go" class="Bool"("DisabledEnum"=T1."Disabled and Grayed Out" ("Disabled")) -> ()  [unwired: 2 in, 2 out]
          }
        }
      }
      event #19 {
        n763 = event-data() -> ()  [unwired: 1 in, 7 out]
        n764 = flat-sequence {
          tunnel: [w1492] -> _
          tunnel: [w1491] -> _
          tunnel: w1480 -> [w1490]
          tunnel: w1479 -> [w1489]
          frame #0 {
            n765 = property on="Reset Z Motor Steps" class="DigNum (strict)"() -> ("Value"=w1493:i32)  [unwired: 2 in, 2 out]
            n766 = Number To Decimal String(number=w1493) -> (decimal integer string=w1494:string)  [unwired: 1 in]
            n767 = call "mDrive Send Command.vi"("error in (no error)"=w1489, "Extra"=w1494, "Command"=T2."Set Current Position", "VISA resource name"=w1490) -> ("error out"=w1491:errorcluster, "VISA resource name out"=w1492:refnum<visa-resource-name>)  [unwired: 3 in, 1 out]
          }
        }
        n768 = flat-sequence {
          tunnel: [w1496] -> w1482
          tunnel: w1483 -> [w1499]
          tunnel: [w1498] -> w1481
          tunnel: w1484 -> [w1497]
          frame #0 {
            n769 = property on="Reset X Motor Steps" class="DigNum (strict)"() -> ("Value"=w1500:i32)  [unwired: 2 in, 2 out]
            n770 = Number To Decimal String(number=w1500) -> (decimal integer string=w1501:string)  [unwired: 1 in]
            n771 = call "mDrive Send Command.vi"("error in (no error)"=w1499, "Extra"=w1501, "Command"=T2."Set Current Position", "VISA resource name"=w1497) -> ("error out"=w1498:errorcluster, "VISA resource name out"=w1496:refnum<visa-resource-name>)  [unwired: 3 in, 1 out]
          }
        }
        n772 = flat-sequence {
          tunnel: w1488 -> [w1506]
          tunnel: w1487 -> [w1505]
          tunnel: [w1504] -> w1486
          tunnel: [w1503] -> w1485
          frame #0 {
            n773 = property on="Reset Y Motor Steps" class="DigNum (strict)"() -> ("Value"=w1507:i32)  [unwired: 2 in, 2 out]
            n774 = Number To Decimal String(number=w1507) -> (decimal integer string=w1508:string)  [unwired: 1 in]
            n775 = call "mDrive Send Command.vi"("error in (no error)"=w1505, "Extra"=w1508, "Command"=T2."Set Current Position", "VISA resource name"=w1506) -> ("error out"=w1503:errorcluster, "VISA resource name out"=w1504:refnum<visa-resource-name>)  [unwired: 3 in, 1 out]
          }
        }
      }
    }
  }
  n776 = flat-sequence {
    tunnel: w6 -> [w1514]
    tunnel: w5 -> [w1511]
    frame #0 {
      n777 = call "mDrive Send Command.vi"("error in (no error)"=w1511, "Command"=T2."Stop", "VISA resource name"=w1514) -> ("error out"=w1512:errorcluster, "VISA resource name out"=w1513:refnum<visa-resource-name>)  [unwired: 4 in, 1 out]
      n778 = VISA Close(VISA resource name=w1513, error in (no error)=w1512) -> ()  [unwired: 1 out]
    }
  }
  n779 = flat-sequence {
    tunnel: w52 -> [w1519]
    tunnel: w51 -> [w1516]
    frame #0 {
      n780 = call "mDrive Send Command.vi"("error in (no error)"=w1516, "Command"=T2."Stop", "VISA resource name"=w1519) -> ("error out"=w1517:errorcluster, "VISA resource name out"=w1518:refnum<visa-resource-name>)  [unwired: 4 in, 1 out]
      n781 = VISA Close(VISA resource name=w1518, error in (no error)=w1517) -> ()  [unwired: 1 out]
    }
  }
  n782 = flat-sequence {
    tunnel: w79 -> [w1524]
    tunnel: w78 -> [w1521]
    frame #0 {
      n783 = call "mDrive Send Command.vi"("error in (no error)"=w1521, "Command"=T2."Stop", "VISA resource name"=w1524) -> ("error out"=w1522:errorcluster, "VISA resource name out"=w1523:refnum<visa-resource-name>)  [unwired: 4 in, 1 out]
      n784 = VISA Close(VISA resource name=w1523, error in (no error)=w1522) -> ()  [unwired: 1 out]
    }
  }
  n785 = flat-sequence {
    tunnel: w2 -> [w1529]
    tunnel: w1 -> [w1526]
    frame #0 {
      n786 = call "mDrive Send Command.vi"("error in (no error)"=w1526, "Command"=T2."Stop", "VISA resource name"=w1529) -> ("error out"=w1527:errorcluster, "VISA resource name out"=w1528:refnum<visa-resource-name>)  [unwired: 4 in, 1 out]
      n787 = VISA Close(VISA resource name=w1528, error in (no error)=w1527) -> ()  [unwired: 1 out]
    }
  }
  "Y COM PORT" <- w82
  "X COM PORT" <- w57
  "Z COM PORT" <- w44
  "R COM PORT" <- w11
